vi "Vision.vi"() -> ()   [LabVIEW 2013]
doc: "Use this template to build a standard state machine design pattern. Each state executes code and determines which state to transition to. Contrast this design pattern with the User Interface Event Handler pattern, in which code executes in response to user actions. Contrast this design pattern also with the Queued Message Handler pattern, in which each message handling code can queue zero or more new messages."
uses:
  StateMachineStates 1.ctl
  <vilib>/DAQmx/write.llb/DAQmx Write (Digital Bool 1Line 1Point).vi
  <vilib>/DAQmx/read.llb/DAQmx Read (Digital Bool 1Line 1Point).vi
  <vilib>/DAQmx/read.llb/DAQmx Read (Counter DBL 1Chan 1Samp).vi
  <vilib>/DAQmx/read.llb/DAQmx Read (Counter U32 1Chan 1Samp).vi
  <vilib>/DAQmx/miscellaneous.llb/DAQmx Fill In Error Info.vi
  <vilib>/DAQmx/create/channels.llb/DAQmx Create Channel (CI-Pulse Width).vi
  <vilib>/DAQmx/create/channels.llb/DAQmx Create Channel (CI-Count Edges).vi
panel:
  in  "Dynamic pump power":bool
  out "Set 4":bool[](array[boolean])
  out "Set 3":bool[](array[boolean])
  out "Set 2":bool[](array[boolean])
  out "Set 1":bool[](array[boolean])
  out "Photon time (ms)":dbl format="%.2f"
  in  "Interval (ms)":u32
  out "Repetition":dbl
  in  "Repetitions":dbl=1.0
  out "WP time (ms)":u32
  out "VISA Handle out":refnum<visa-resource-name>="ASRL5::INSTR"
  out "Initializing":bool
  out "Trial mode":T1(ring)
  in  "Frequency of LED trials\nfor Mixed mode":dbl=30.0
  out "Bright trial\nrequested":bool
  out "Observer Ready":bool
  in  "Bright/mixed mode \nLED voltage (V)":dbl=2.6 min=-3.0 max=4.0 format="%.2f"
  in  "Manual voltage (V)":dbl=2.6 format="%.2p"
  in  "GPIB address":string="15"
  in  "Period (ms)":i64=20
  in  "Pulse length (ms)":dbl=50.0
  out "L/R WP":dbl format="%.2f"
  in  "Manually \ninitialize":bool
  in  "COM for WPs":u8=3
  in  "L/R control method":enum16{"Liquid crystal", "Motorized waveplate"}(ring)=enum."Motorized waveplate"
  out "Blocked trial #":i32
  in  "Manual photon #":i32
  out "Photon #":i32
  out "LED Voltage":dbl
  in  "Blocking requirements":cluster{"Value":dbl, " Number":i32}[](array[cluster])
  in  "Manual":bool
  in  "Path":path=path "C:/Users/Lab/Dropbox/Vision software/Data"
  out "Counts 2":u32
  out "Counts 1":u32
  in  "Delay for APDs (ms)":u32=25
  in  "Counter 2":tag="Dev1/ctr1"
  in  "Counter 1":tag="Dev1/ctr0"
  out "Trial #":i32
  in  "Mode":T2(ring)=enum."Mixed"
  in  "Audio":bool=TRUE
  in  "Self-paced":bool
  out "Stimulus":bool
  out "Location Set":bool
  out "Stimulus \nlocation":string
  out "Waiting":bool
  out "Observer Responded":bool
  out "Response \ntime (ms)":dbl
  out "Observer \nchoice":string
  out "Confidence":i32
  in  "stop":bool
  in  "Next Trial":bool
  in  "Create New File":bool
  out "Subject #":string
  # "Settings for Blocking\nand Mixed Mode"
  # "Instructions: Run VI. Enter blocking requirements, then press\nCreate New File. Initialize waveplates if necessary, and set\nhighlighted controls to desired values. Press Next Trial to begin."
  # "Researcher Interface"
  # "Trial Options"
  # "Counter Options\n(same for LED &\ndetector tests)"
  # "Trial Information"
  # "Enter pre-set blocking \nrequirements\nbefore creating a new file."
  # "Troubleshooting"
  # "Photon Options"
  # "LED Options"
  # "Waveplates"
  # "Status"
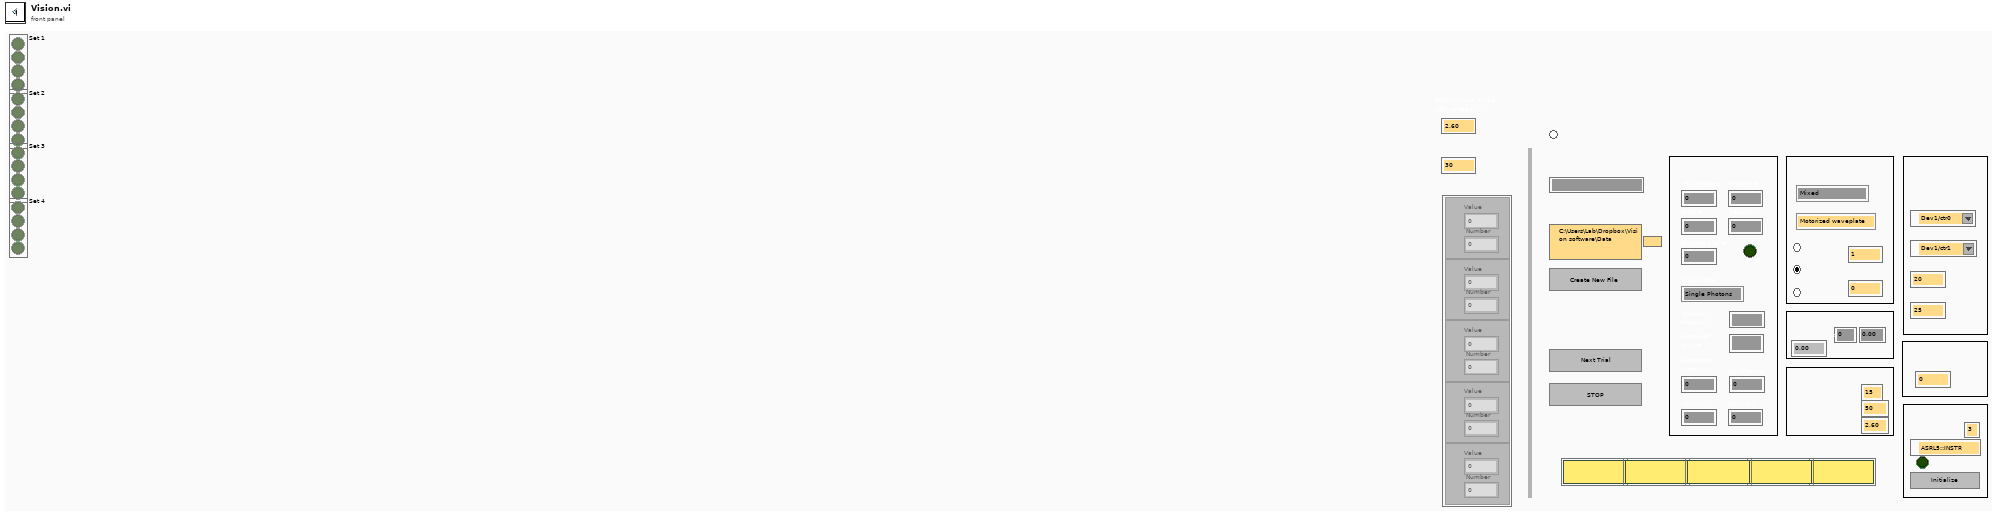
[diagram p1: front panel]
types:
  T1 = enum16{"Single Photons", "Detector Tests", "LED", "Mixed LED"}
  T2 = enum16{"Single Photons", "Detector Tests", "LED", "Mixed"}
  T3 = typedef "StateMachineStates 1.ctl" = enum16{"WaitResearcher", "SetWP", "SetLC", "WaitObserverReady", "Photons", "Detectors", "LED", "WaitObserverResponse", "CleanUp", "Stop"}
  T4 = enum16{"0", "1", "2", "3", "4", "5", "6", "7", "8", "9", "A", "B", "C", "D", "E", "F", "G", "H", "I", "J", "K", "L", "M", "N", "O", "P", "Q", "R", "S", "T", "U", "V", "W", "X", "Y", "Z", "F1", "F2", "F3", "F4", "F5", "F6", "F7", "F8", "F9", "F10", "F11", "F12", "F13", "F14", "F15", "ADD", "BACK", "BACKSLASH", "CAPITAL", "COMMA", "DECIMAL", "DELETE", "DIVIDE", "DOWN", "END", "EQUALS", "ESCAPE", "GRAVE (`)", "HOME", "INSERT", "LBRACKET", "LCONTROL", "LEFT", "L ALT", "LSHIFT", "LWIN", "MINUS", "MULTIPLY", "NEXT", "NUMLOCK", "NUMPAD_0", "NUMPAD_1", "NUMPAD_2", "NUMPAD_3", "NUMPAD_4", "NUMPAD_5", "NUMPAD_6", "NUMPAD_7", "NUMPAD_8", "NUMPAD_9", "PAUSE", "PERIOD", "PRIOR (PG UP)", "RBRACKET", "RCONTROL", "RETURN", "RIGHT", "R ALT", "RSHIFT", "RWIN", "SCROLL", "SEMICOLON", "SLASH", "SPACE", "SUBTRACT", "TAB", "UP", "ENTER (num pad)", "' (quote)"}
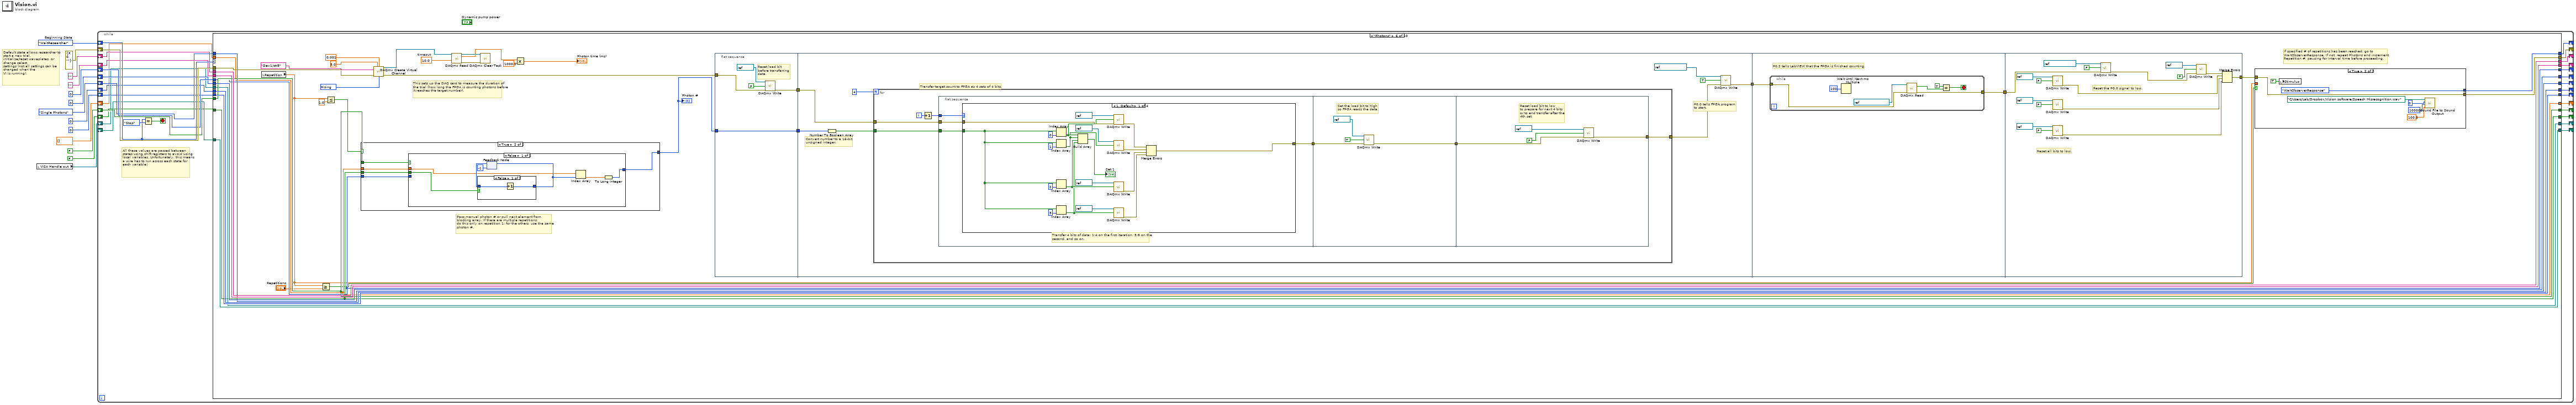
[diagram p0: block diagram]
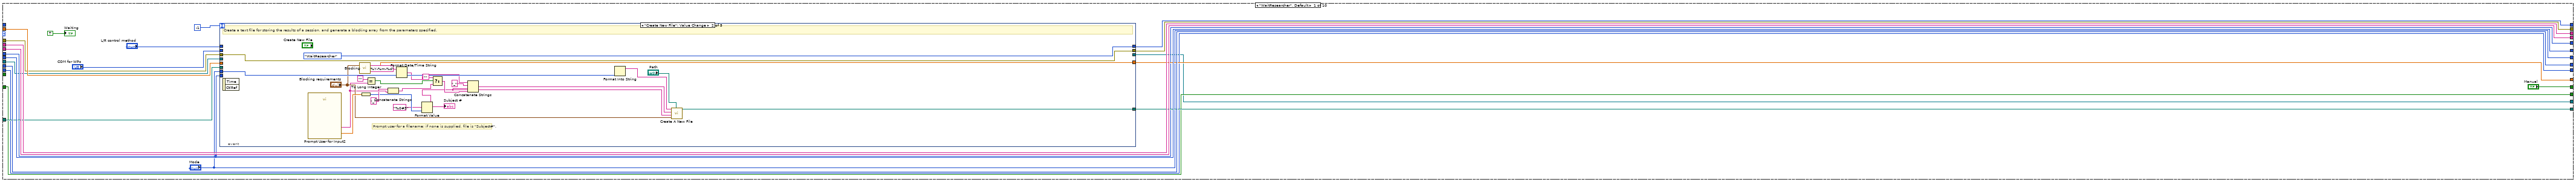
[diagram p2: hidden frame]
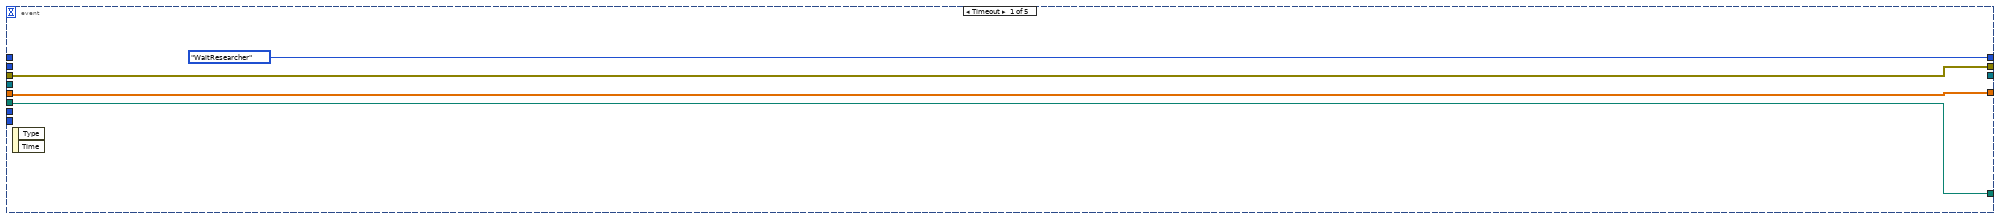
[diagram p3: hidden frame]
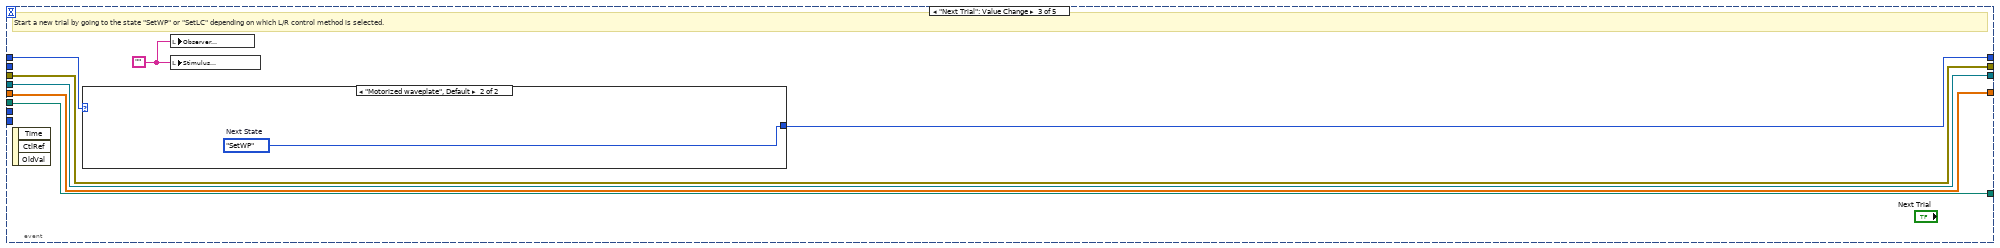
[diagram p4: hidden frame]
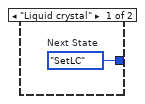
[diagram p5: hidden frame]
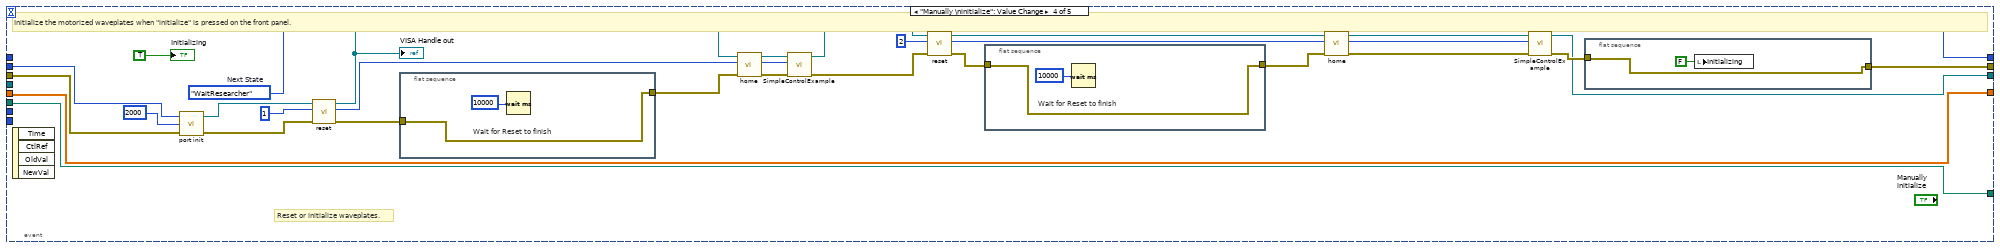
[diagram p6: hidden frame]
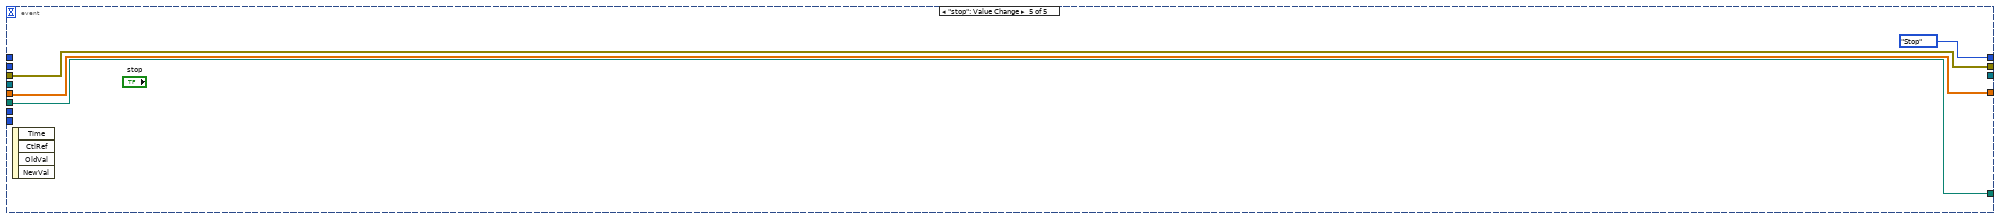
[diagram p7: hidden frame]
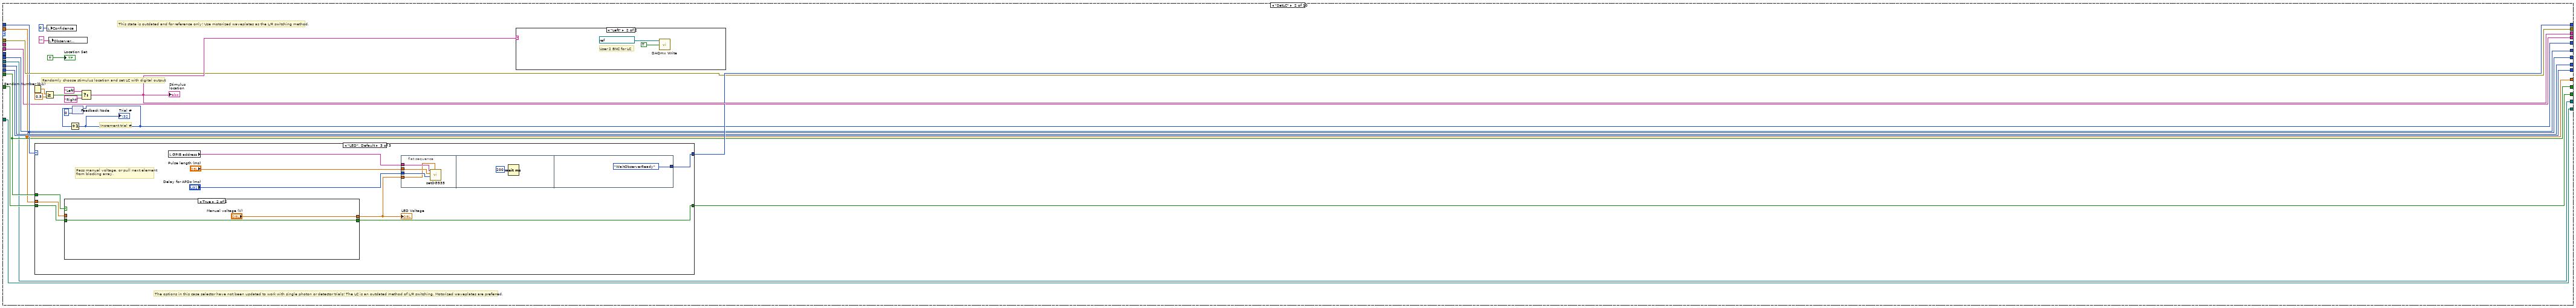
[diagram p8: hidden frame]
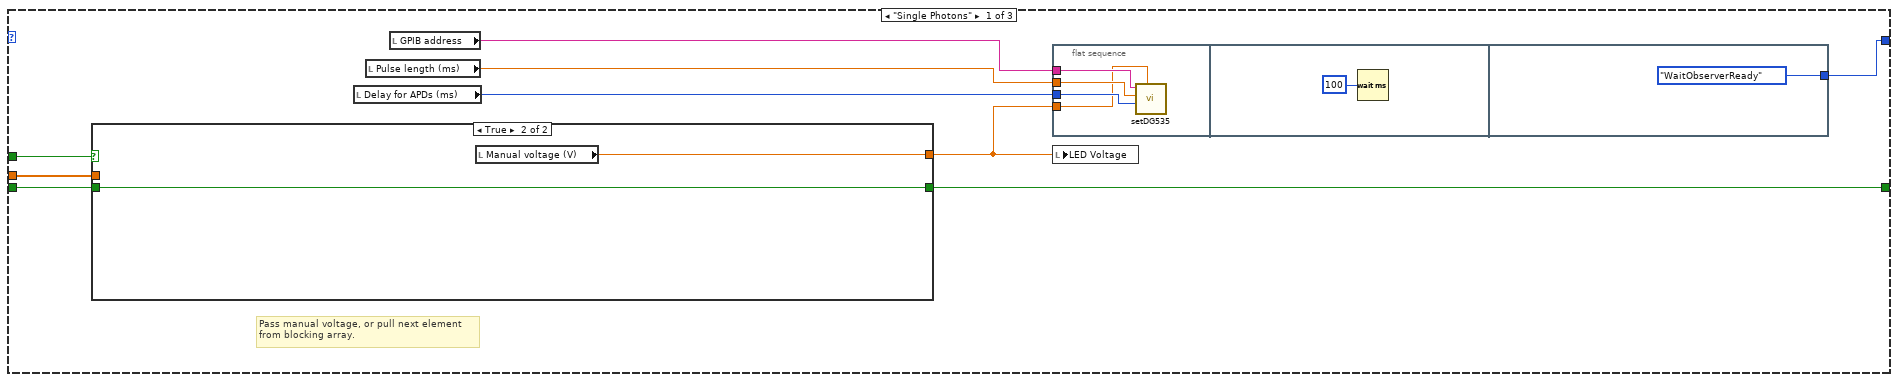
[diagram p9: hidden frame]
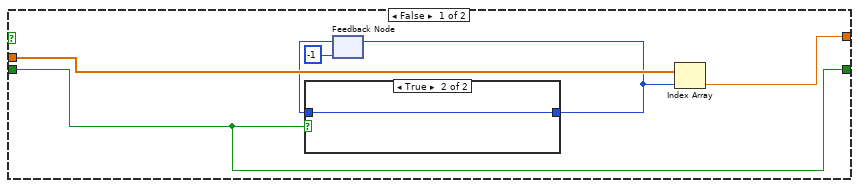
[diagram p10: hidden frame]
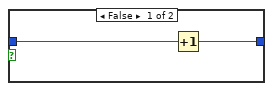
[diagram p11: hidden frame]
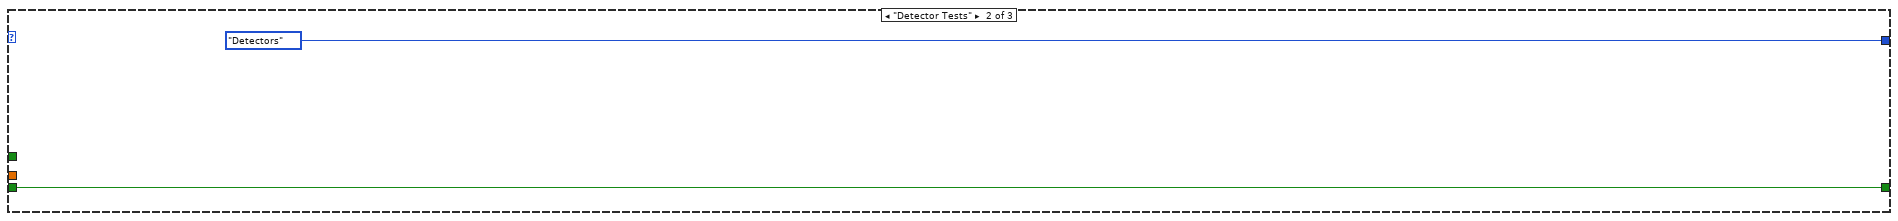
[diagram p12: hidden frame]
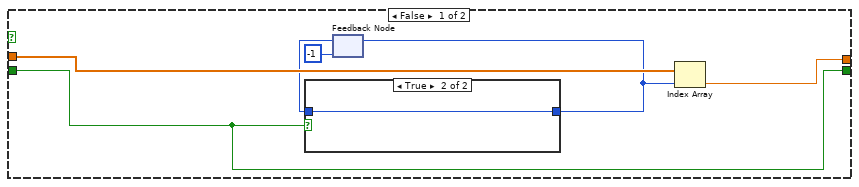
[diagram p13: hidden frame]
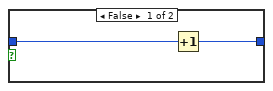
[diagram p14: hidden frame]
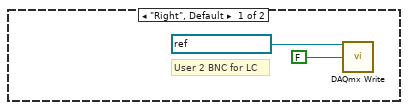
[diagram p15: hidden frame]
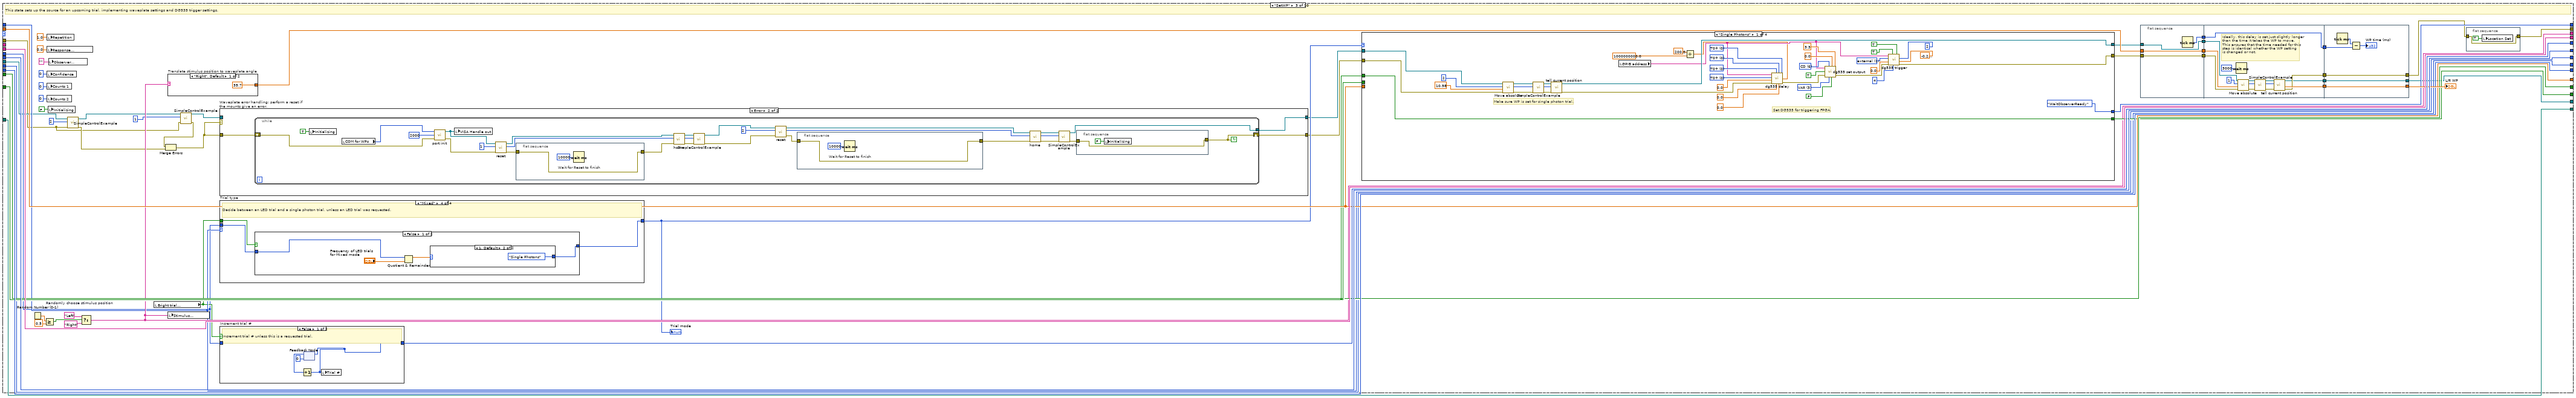
[diagram p16: hidden frame]
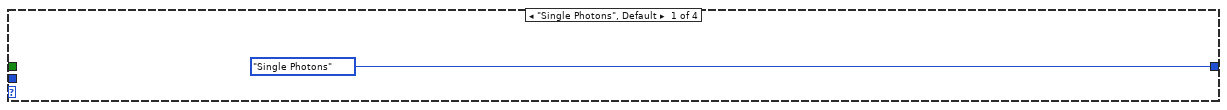
[diagram p19: hidden frame]
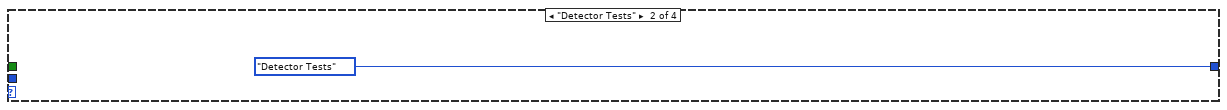
[diagram p20: hidden frame]
diagram:
  w13 = StateMachineStates_1."WaitResearcher"  # Beginning State
  # "Default state allows researcher to start a new trial,\ninitialize/reset waveplates, or change select\nsettings (not all settings can be changed when the\nVI is running)."
  n1 = local read "VISA Handle out"() -> (w1:refnum<visa-resource-name>)
  n2 = while {
    shift-right: [w40] -> _
    shift-left: w13 -> [w41]
    shift-right: [w19] -> _
    shift-left: errorcluster {"status"=FALSE, "code"=0, "source"=""} ("error out") -> [w39]
    shift-right: [w38] -> _
    shift-left: "" -> [w37]
    shift-right: [w36] -> _
    shift-left: "" ("Observer choice") -> [w35]
    shift-right: [w34] -> _
    shift-left: 0 -> [w33]
    shift-right: [w32] -> _
    shift-left: 0 ("Confidence") -> [w31]
    shift-right: [w30] -> _
    shift-left: T2."Single Photons" ("Mode") -> [w29]
    shift-right: [w28] -> _
    shift-left: u32 0 ("Counts 1") -> [w14]
    shift-right: [w27] -> _
    shift-left: u32 0 ("Counts 2") -> [w26]
    shift-right: [w25] -> _
    shift-left: _ -> [w24]
    shift-right: [w23] -> _
    shift-left: dbl[] [] ("Blocking array") -> [w22]
    shift-right: [w21] -> _
    shift-left: FALSE ("Manual") -> [w20]
    shift-right: [w18] -> _
    shift-left: FALSE ("Bright trial\nrequested") -> [w17]
    shift-right: [w16] -> _
    shift-left: w1 -> [w15]
    stop <- w43 stop-if-true
    # "All these values are passed between states using shift registers to avoid using local variables. Unfortunately, this means a wire has to run across each state for each variable!"
    n3 = Equal?(x=w41, y=StateMachineStates_1."Stop" ("States")) -> (x = y?=w43:bool)
    n4 = case shown="\"Photons\"" w41 {
      selector: w41 -> [_ _ _ w527 _ _ _ _ _ _]
      tunnel: [w65 w160 w268 w528 StateMachineStates_1."WaitObserverResponse" ("Next State") w648 w838 w945 w1014 w1092] -> w40
      tunnel: [w50 w157 w267 w516 w607 w638 w824 w949 w997 w1097] -> w19
      tunnel: w39 -> [w51 w157 w226 w517 w593 w625 w840 w949 w991 w1096]
      tunnel: [w64 w161 w261 w531 w608 w651 w846 w951 w1010 w1108] -> w38
      tunnel: w37 -> [w64 _ _ w531 w608 w651 w846 w951 w1010 w1108]
      tunnel: [w63 w145 w278 w530 w611 w650 w819 w946 w1009 w1107] -> w36
      tunnel: w35 -> [w63 w145 w278 w530 w611 w650 _ _ w1009 w1107]
      tunnel: [w53 w151 w276 w529 w598 w641 w841 w950 w1001 w1106] -> w34
      tunnel: w33 -> [w53 _ w242 w529 w598 w641 w841 w950 w1001 w1106]
      tunnel: [w62 w158 w277 w526 w610 w649 w821 w944 w1013 w1105] -> w32
      tunnel: w31 -> [w62 w158 w277 w526 w610 w649 w821 _ w1013 w1105]
      tunnel: ["Mode" w150 w257 w524 w603 w647 w823 w943 w1008 w1104] -> w30
      tunnel: w29 -> [_ w150 w257 w523 w603 w647 w823 w943 w1008 w1104]
      tunnel: [w59 w154 w260 w522 w602 w646 w822 w942 w1006 w1103] -> w28
      tunnel: [w52 w153 w273 w521 w601 w645 w820 w941 w1007 w1102] -> w27
      tunnel: w14 -> [w59 w154 w260 w522 _ w646 _ w942 w1006 w1103]
      tunnel: w26 -> [w52 w153 w273 w521 _ w645 _ w941 w1007 w1102]
      tunnel: [w58 w152 w274 w520 w600 w644 w845 w940 w1005 w1101] -> w25
      tunnel: w24 -> [w57 w152 w274 w520 w600 w644 w845 w940 w1005 w1101]
      tunnel: [w56 w148 w272 w519 w599 w642 w842 w939 w1003 w1100] -> w23
      tunnel: w22 -> [w55 w148 w272 w519 w599 w642 w842 w939 w1003 w1100]
      tunnel: ["Manual" w149 w270 w518 w597 w643 w843 w938 w998 w1099] -> w21
      tunnel: w20 -> [_ w149 w270 w518 w597 w643 w843 w938 w995 w1099]
      tunnel: [w47 w146 w269 w514 w592 w639 w836 w937 w993 w1098] -> w18
      tunnel: w17 -> [w47 w147 w271 w514 w592 w639 w836 w937 _ w1098]
      tunnel: [w46 w142 w254 w513 w591 w640 w835 w936 w992 w1095] -> w16
      tunnel: w15 -> [w44 w142 w235 w513 w591 w640 w835 w936 w992 w1095]
      frame "WaitResearcher", Default {
        n5 = event shown="[1] \"Create New File\": Value Change" {
          selector: _ -> [_ _ _ _ _]
          dyn-events: _ -> [_ _ _ _ _]
          timeout: -1 -> [_ _ _ _ _]
          tunnel: [StateMachineStates_1."WaitResearcher" ("Next State") StateMachineStates_1."WaitResearcher" ("Next State") w96 w131 StateMachineStates_1."Stop" ("Next State")] -> w65
          tunnel: "Mode" -> [_ w88 _ _ _]
          tunnel: [w69 w82 w98 w130 w140] -> w58
          tunnel: w57 -> [w69 _ w98 w130 w140]
          tunnel: [w68 w86 w97 w118 w139] -> w56
          tunnel: w55 -> [w68 _ w97 w118 w139]
          tunnel: w53 -> [_ _ _ _ _]
          tunnel: w51 -> [w67 w81 w94 w119 w138]
          tunnel: [w67 w81 w94 w108 w138] -> w50
          tunnel: "L/R control method" -> [_ _ w95 _ _]
          tunnel: "COM for WPs" -> [_ _ _ w106 _]
          tunnel: [_ _ w93 w104 _] -> w46
          tunnel: w44 -> [_ _ w93 _ _]
          event Timeout {
            n6 = event-data() -> ()  [unwired: 1 in, 2 out]
          }
          event "Create New File": Value Change {
            # "Prompt user for a filename; if none is supplied, file is \"Subject#\"."
            # "Create a text file for storing the results of a session, and generate a blocking array from the parameters specified."
            n7 = event-data() -> ()  [unwired: 1 in, 2 out]
            n8 = call "Prompt User for Input2"() -> ("Subject #"=w91:dbl, "Filename"=w76:string)  [unwired: 16 in, 2 out]
            n9 = call "Blocking.vi"("Blocking requirements"="Blocking requirements") -> ("Blocking array"=w86:dbl[])  [unwired: 2 in]
            n10 = To Long Integer(number=w91) -> (32bit integer=w72:i32)
            n11 = Equal?(x="", y=w76) -> (x = y?=w89:bool)
            n12 = Concatenate Strings("_" ("string"), w76) -> (w79:string)
            n13 = Format Date/Time String(time format string (%c)="%Y-%m-%d") -> (date/time string=w77:string)  [unwired: 2 in]
            n14 = Format Value(format string="%0#3", value (0)=w72) -> (output string=w71:string)  [unwired: 1 in]
            "Subject #" <- w71
            n15 = Select(t="", s=w89, f=w79) -> (s? t:f=w74:string)
            n16 = Concatenate Strings(w77, "_" ("string"), w71, w74) -> (w83:string)
            n17 = Format Into String(w88) -> (resulting string=w87:string)  [unwired: 3 in, 1 out]
            n18 = call "Create A New File.vi"("Path in"="Path", "Blocking requirements"="Blocking requirements", "Subject #"=w71, "Filename"=w83, "Mode"=w87) -> ("Path out"=w82:path)  [unwired: 6 in]
          }
          event "Next Trial": Value Change {
            w99 = ""
            # "Start a new trial by going to the state \"SetWP\" or \"SetLC\" depending on which L/R control method is selected."
            n19 = event-data() -> ()  [unwired: 1 in, 3 out]
            n20 = case shown="\"Motorized waveplate\", Default" w95 {
              tunnel: [w100 w101] -> w96
              frame "Liquid crystal" {
                w100 = StateMachineStates_1."SetLC"  # Next State
              }
              frame "Motorized waveplate", Default {
                w101 = StateMachineStates_1."SetWP"  # Next State
              }
            }
            n21 = local write "Observer \nchoice"(w99) -> ()
            n22 = local write "Stimulus \nlocation"(w99) -> ()
          }
          event "Manually \ninitialize": Value Change {
            w131 = StateMachineStates_1."WaitResearcher"  # Next State
            # "Reset or initialize waveplates."
            # "Initialize the motorized waveplates when \"initialize\" is pressed on the front panel."
            n23 = event-data() -> ()  [unwired: 1 in, 4 out]
            n24 = call "port init.vi"("error in"=w119, "Timeout (ms)"=u32 2000 ("Timeout (300 ms)"), "SerialPort"=w106) -> ("error out"=w126:errorcluster, "Visa Handle"=w125:refnum<visa-resource-name>)  [unwired: 1 in]
            n25 = call "reset.vi"("error in"=w126, "Axis in"=1, "VISA Handle in"=w125) -> ("error out"=w123:errorcluster, "Axis out"=w124:i32, "VISA Handle out"=w102:refnum<visa-resource-name>)  [unwired: 3 in, 1 out]
            "VISA Handle out" <- w102
            n26 = flat-sequence {
              tunnel: [w136] -> w122
              tunnel: w123 -> [w136]
              frame #0 {
                # "Wait for Reset to finish"
                n27 = Wait (ms)(milliseconds to wait=u32 10000) -> ()  [unwired: 1 out]
              }
            }
            n28 = call "home.vi"("error in"=w122, "Axis in"=w124, "VISA Handle in"=w102) -> ("error out"=w128:errorcluster, "Axis out"=w127:i32, "VISA Handle out"=w129:refnum<visa-resource-name>)  [unwired: 3 in, 1 out]
            n29 = call "SimpleControlExample.vi"("error in"=w128, "Axis in"=w127, "VISA Handle in"=w129) -> ("error out"=w107:errorcluster, "VISA Handle out"=w105:refnum<visa-resource-name>)  [unwired: 3 in, 2 out]
            n30 = call "reset.vi"("error in"=w107, "Axis in"=2, "VISA Handle in"=w105) -> ("error out"=w113:errorcluster, "Axis out"=w114:i32, "VISA Handle out"=w110:refnum<visa-resource-name>)  [unwired: 3 in, 1 out]
            n31 = flat-sequence {
              tunnel: [w134] -> w112
              tunnel: w113 -> [w134]
              frame #0 {
                # "Wait for Reset to finish"
                n32 = Wait (ms)(milliseconds to wait=u32 10000) -> ()  [unwired: 1 out]
              }
            }
            n33 = call "home.vi"("error in"=w112, "Axis in"=w114, "VISA Handle in"=w110) -> ("error out"=w116:errorcluster, "Axis out"=w115:i32, "VISA Handle out"=w117:refnum<visa-resource-name>)  [unwired: 3 in, 1 out]
            n34 = call "SimpleControlExample.vi"("error in"=w116, "Axis in"=w115, "VISA Handle in"=w117) -> ("error out"=w109:errorcluster, "VISA Handle out"=w104:refnum<visa-resource-name>)  [unwired: 3 in, 2 out]
            n35 = flat-sequence {
              tunnel: w109 -> [w133]
              tunnel: [w133] -> w108
              frame #0 {
                n36 = local write "Initializing"(FALSE ("Initializing waveplates")) -> ()
              }
            }
            "Initializing" <- TRUE ("Initializing waveplates")
          }
          event "stop": Value Change {
            n37 = event-data() -> ()  [unwired: 1 in, 4 out]
          }
        }
        "Waiting" <- TRUE ("Waiting")
      }
      frame "SetLC" {
        # "This state is outdated and for reference only! Use motorized waveplates as the L/R switching method."
        # "The options in this case selector have not been updated to work with single photon or detector trials! The LC is an outdated method of L/R switching. Motorized waveplates are preferred."
        # "Randomly choose stimulus location and set LC with digital output"
        # "Increment trial #"
        n38 = Random Number (0-1)() -> (number: 0 to 1=w166:dbl)
        n39 = case shown="\"LED\", Default" w150 {
          tunnel: [w172 StateMachineStates_1."Detectors" ("Next State") w197] -> w160
          tunnel: w149 -> [w175 _ w203]
          tunnel: w148 -> [w174 _ w202]
          tunnel: w147 -> [w171 w193 w196]
          tunnel: [w170 w193 w195] -> w146
          frame "Single Photons" {
            # "Pass manual voltage, or pull next element\nfrom blocking array."
            n40 = case shown="True" w175 {
              tunnel: [w186 w191] -> w167
              tunnel: w174 -> [w187 _]
              tunnel: w171 -> [w182 w192]
              tunnel: [w182 w192] -> w170
              frame False {
                n41 = feedback #1(-1 ("x+1")) -> (w185:i32)
                n42 = case shown="True" w182 {
                  tunnel: w185 -> [w189 w190]
                  tunnel: [w188 w190] -> w183
                  frame False {
                    n43 = Increment(x=w189) -> (x+1=w188:i32)
                  }
                  frame True {
                  }
                }
                n44 = feedback-in #1(w183) -> ()
                n45 = Index Array(array=w187, index=w183) -> (element=w186:dbl)
              }
              frame True {
                n46 = local read "Manual voltage (V)"() -> (w191:dbl)
              }
            }
            n47 = local read "Delay for APDs (ms)"() -> (w169:u32)
            n48 = local read "Pulse length (ms)"() -> (w168:dbl)
            n49 = local read "GPIB address"() -> (w173:string)
            n50 = flat-sequence {
              tunnel: w169 -> [w179]
              tunnel: w173 -> [w178]
              tunnel: w168 -> [w177]
              tunnel: w167 -> [w176]
              tunnel: [StateMachineStates_1."WaitObserverReady" ("Next State")] -> w172
              frame #0 {
                n51 = call "setDG535.vi"("amplitude"=w176, "Delay (ms)"=w179, "Pulse length (ms)"=w177, "GPIB address"=w178) -> ()  [unwired: 7 in, 1 out]
              }
              frame #1 {
                n52 = Wait (ms)(milliseconds to wait=u32 100) -> ()  [unwired: 1 out]
              }
              frame #2 {
              }
            }
            n53 = local write "LED Voltage"(w167) -> ()
          }
          frame "Detector Tests" {
          }
          frame "LED", Default {
            # "Pass manual voltage, or pull next element\nfrom blocking array."
            n54 = case shown="True" w203 {
              tunnel: [w214 "Manual voltage (V)"] -> w198
              tunnel: w202 -> [w215 _]
              tunnel: w196 -> [w210 w219]
              tunnel: [w210 w219] -> w195
              frame False {
                n55 = feedback #2(-1 ("x+1")) -> (w213:i32)
                n56 = case shown="True" w210 {
                  tunnel: w213 -> [w217 w218]
                  tunnel: [w216 w218] -> w211
                  frame False {
                    n57 = Increment(x=w217) -> (x+1=w216:i32)
                  }
                  frame True {
                  }
                }
                n58 = feedback-in #2(w211) -> ()
                n59 = Index Array(array=w215, index=w211) -> (element=w214:dbl)
              }
              frame True {
              }
            }
            "LED Voltage" <- w198
            n60 = local read "GPIB address"() -> (w200:string)
            n61 = flat-sequence {
              tunnel: "Delay for APDs (ms)" -> [w207]
              tunnel: w200 -> [w206]
              tunnel: "Pulse length (ms)" -> [w205]
              tunnel: w198 -> [w204]
              tunnel: [StateMachineStates_1."WaitObserverReady" ("Next State")] -> w197
              frame #0 {
                n62 = call "setDG535.vi"("amplitude"=w204, "Delay (ms)"=w207, "Pulse length (ms)"=w205, "GPIB address"=w206) -> ()  [unwired: 7 in, 1 out]
              }
              frame #1 {
                n63 = Wait (ms)(milliseconds to wait=u32 200) -> ()  [unwired: 1 out]
              }
              frame #2 {
              }
            }
          }
        }
        n64 = Greater Or Equal?(x=w166, y=0.5) -> (x >= y?=w164:bool)
        n65 = local write "Confidence"(0 ("Confidence")) -> ()
        n66 = local write "Observer \nchoice"("" ("Observer choice")) -> ()
        n67 = feedback #3(0 ("x+1")) -> (w156:i32)
        n68 = Increment(x=w156) -> (x+1=w151:i32)
        "Trial #" <- w151
        n69 = feedback-in #3(w151) -> ()
        n70 = Select(t="Left", s=w164, f="Right") -> (s? t:f=w161:string)
        "Stimulus \nlocation" <- w161
        n71 = case shown="\"Left\"" w161 {
          frame "Right", Default {
            # "User 2 BNC for LC"
            n72 = call-poly <vilib>:"DAQmx Write.vi"("task/channels in"=refnum<k21> "LC_Controller", "data"=FALSE) -> ()  [unwired: 11 in, 3 out]
          }
          frame "Left" {
            # "User 2 BNC for LC"
            n73 = call-poly <vilib>:"DAQmx Write.vi"("task/channels in"=refnum<k21> "LC_Controller", "data"=TRUE) -> ()  [unwired: 11 in, 3 out]
          }
        }
        "Location Set" <- TRUE ("LC Set")
      }
      frame "SetWP" {
        # "This state sets up the source for an upcoming trial, implementing waveplate settings and DG535 trigger settings."
        n74 = Random Number (0-1)() -> (number: 0 to 1=w262:dbl)
        n75 = Greater Or Equal?(x=w262, y=0.5) -> (x >= y?=w264:bool)
        n76 = local write "Repetition"(1.0 ("Repitition #")) -> ()
        n77 = local write "Response \ntime (ms)"(0.0 ("Response \ntime (ms)")) -> ()
        n78 = local write "Confidence"(0 ("Confidence")) -> ()
        n79 = local write "Counts 1"(u32 0 ("Counts 1")) -> ()
        n80 = local write "Counts 2"(u32 0 ("Counts 2")) -> ()
        n81 = local write "Initializing"(FALSE ("Initializing waveplates")) -> ()
        n82 = local write "Observer \nchoice"("" ("Observer \nchoice")) -> ()
        n83 = call "SimpleControlExample.vi"("error in"=w226, "Axis in"=2, "VISA Handle in"=w235) -> ("error out"=w227:errorcluster, "VISA Handle out"=w233:refnum<visa-resource-name>)  [unwired: 3 in, 2 out]
        n84 = Select "Randomly choose stimulus position"(t="Left", s=w264, f="Right") -> (s? t:f=w261:string)
        n85 = local read "Bright trial\nrequested"() -> (w243:bool)
        n86 = case "Translate stimulus position to waveplate angle" shown="\"Right\", Default" w261 {
          tunnel: [35.7 ("New target position (units)") 80.7 ("New target position (units)")] -> w258
          frame "Right", Default {
          }
          frame "Left" {
          }
        }
        n87 = local write "Stimulus \nlocation"(w261) -> ()
        n88 = call "SimpleControlExample.vi"("error in"=w226, "Axis in"=1, "VISA Handle in"=w233) -> ("error out"=w228:errorcluster, "VISA Handle out"=w231:refnum<visa-resource-name>)  [unwired: 3 in, 2 out]
        n89 = Merge Errors(w228, w227) -> (w225:errorcluster)
        n90 = case "Waveplate error handling: perform a reset if the mounts give an error." shown="Error" w225 {
          tunnel: w225 -> [w280 w283]
          tunnel: [w280 w281] -> w229
          tunnel: [w279 w282] -> w230
          tunnel: w231 -> [w279 _]
          frame No Error {
          }
          frame Error {
            n91 = while {
              tunnel: [w286] -> w282
              shift-right: [w284] -> w281
              shift-left: w283 -> [w289]
              stop <- w284 continue-if-true
              n92 = local write "Initializing"(TRUE ("Initializing waveplates")) -> ()
              n93 = local read "COM for WPs"() -> (w288:u8)
              n94 = call "port init.vi"("error in"=w289, "Timeout (ms)"=u32 2000 ("Timeout (300 ms)"), "SerialPort"=w288) -> ("error out"=w307:errorcluster, "Visa Handle"=w287:refnum<visa-resource-name>)  [unwired: 1 in]
              n95 = local write "VISA Handle out"(w287) -> ()
              n96 = call "reset.vi"("error in"=w307, "Axis in"=1, "VISA Handle in"=w287) -> ("error out"=w305:errorcluster, "Axis out"=w306:i32, "VISA Handle out"=w290:refnum<visa-resource-name>)  [unwired: 3 in, 1 out]
              n97 = flat-sequence {
                tunnel: [w315] -> w304
                tunnel: w305 -> [w315]
                frame #0 {
                  # "Wait for Reset to finish"
                  n98 = Wait (ms)(milliseconds to wait=u32 10000) -> ()  [unwired: 1 out]
                }
              }
              n99 = call "home.vi"("error in"=w304, "Axis in"=w306, "VISA Handle in"=w290) -> ("error out"=w309:errorcluster, "Axis out"=w308:i32, "VISA Handle out"=w310:refnum<visa-resource-name>)  [unwired: 3 in, 1 out]
              n100 = call "SimpleControlExample.vi"("error in"=w309, "Axis in"=w308, "VISA Handle in"=w310) -> ("error out"=w292:errorcluster, "VISA Handle out"=w291:refnum<visa-resource-name>)  [unwired: 3 in, 2 out]
              n101 = call "reset.vi"("error in"=w292, "Axis in"=2, "VISA Handle in"=w291) -> ("error out"=w297:errorcluster, "Axis out"=w298:i32, "VISA Handle out"=w294:refnum<visa-resource-name>)  [unwired: 3 in, 1 out]
              n102 = flat-sequence {
                tunnel: [w313] -> w296
                tunnel: w297 -> [w313]
                frame #0 {
                  # "Wait for Reset to finish"
                  n103 = Wait (ms)(milliseconds to wait=u32 10000) -> ()  [unwired: 1 out]
                }
              }
              n104 = call "home.vi"("error in"=w296, "Axis in"=w298, "VISA Handle in"=w294) -> ("error out"=w300:errorcluster, "Axis out"=w299:i32, "VISA Handle out"=w301:refnum<visa-resource-name>)  [unwired: 3 in, 1 out]
              n105 = call "SimpleControlExample.vi"("error in"=w300, "Axis in"=w299, "VISA Handle in"=w301) -> ("error out"=w293:errorcluster, "VISA Handle out"=w286:refnum<visa-resource-name>)  [unwired: 3 in, 2 out]
              n106 = flat-sequence {
                tunnel: w293 -> [w312]
                tunnel: [w312] -> w284
                frame #0 {
                  n107 = local write "Initializing"(FALSE ("Initializing waveplates")) -> ()
                }
              }
            }
          }
        }
        n108 = case "Trial type" shown="\"Mixed\"" w257 {
          tunnel: [T1."Single Photons" ("Mode") T1."Detector Tests" ("Mode") T1."LED" ("Mode") w325] -> w256
          tunnel: w242 -> [_ _ _ w326]
          tunnel: w243 -> [_ _ _ w324]
          frame "Single Photons", Default {
          }
          frame "Detector Tests" {
          }
          frame "LED" {
          }
          frame "Mixed" {
            # "Decide between an LED trial and a single photon trial, unless an LED trial was requested."
            n109 = case shown="False" w324 {
              tunnel: w326 -> [w330 _]
              tunnel: [w327 T1."Mixed LED" ("Mode")] -> w325
              frame False {
                n110 = Quotient & Remainder(x=w330, y="Frequency of LED trials\nfor Mixed mode") -> (x-y*floor(x/y)=w328:dbl)  [unwired: 1 out]
                n111 = case shown="1, Default" w328 {
                  tunnel: [T1."Mixed LED" ("Mode") T1."Single Photons" ("Mode")] -> w327
                  frame 0 {
                  }
                  frame 1, Default {
                  }
                }
              }
              frame True {
              }
            }
          }
        }
        "Trial mode" <- w256
        n112 = case "Increment trial #" shown="False" w243 {
          tunnel: [w317 w320] -> w276
          tunnel: w242 -> [_ w320]
          frame False {
            # "Increment trial # unless this is a requested trial."
            n113 = feedback #4(0 ("x+1")) -> (w319:i32)
            n114 = Increment(x=w319) -> (x+1=w317:i32)
            n115 = feedback-in #4(w317) -> ()
            n116 = local write "Trial #"(w317) -> ()
          }
          frame True {
          }
        }
        n117 = case shown="\"Single Photons\"" w256 {
          tunnel: [StateMachineStates_1."WaitObserverReady" ("Next State") StateMachineStates_1."Detectors" ("Next State") w462 w502] -> w268
          tunnel: w270 -> [w403 _ w465 _]
          tunnel: w272 -> [_ _ w464 _]
          tunnel: w271 -> [_ w443 w461 w488]
          tunnel: [w403 w443 w460 w488] -> w269
          tunnel: w229 -> [w395 w435 w449 w492]
          tunnel: [w365 w404 w448 w483] -> w252
          tunnel: w230 -> [w364 w433 w446 w490]
          tunnel: [w393 w432 w445 w489] -> w253
          frame "Single Photons" {
            w381 = u32 1 items=["internal", "external", "single shot", "burst", "line"] ("trigger")
            w383 = 3 items=["TTL", "NIM", "ECL", "VAR"] ("mode")
            w385 = u16 6 items=["T0", "A", "B", "AB", "C", "D", "CD"] ("output")
            w388 = u32 0 items=["T0+", "A+", "B+", "C+"] ("D=")
            w389 = u32 0 items=["T0+", "A+", "B+", "D+"] ("C=")
            w390 = u32 0 items=["T0+", "A+", "C+", "D+"] ("B=")
            w391 = u32 0 items=["T0+", "B+", "C+", "D+"] ("A=")
            # "Set DG535 for triggering FPGA."
            # "Make sure WP is set for single photon trial."
            n118 = call "Move absolute.vi"("error in"=w395, "New target position (units)"=10.98, "Axis in"=2, "VISA Handle in"=w364) -> ("error out"=w397:errorcluster, "Axis out"=w398:i32, "VISA Handle out"=w399:refnum<visa-resource-name>)  [unwired: 2 in, 1 out]
            n119 = call "SimpleControlExample.vi"("error in"=w397, "Axis in"=w398, "VISA Handle in"=w399) -> ("error out"=w400:errorcluster, "Axis out"=w401:i32, "VISA Handle out"=w402:refnum<visa-resource-name>)  [unwired: 3 in, 1 out]
            n120 = call "tell current position.vi"("error in"=w400, "Axis in"=w401, "VISA Handle in"=w402) -> ("error out"=w366:errorcluster, "VISA Handle out"=w393:refnum<visa-resource-name>)  [unwired: 2 in, 3 out]
            n121 = local read "GPIB address"() -> (w373:string)
            n122 = Divide(x=200.0 ("D"), y=1000000000.0) -> (x/y=w367:dbl)
            n123 = call "dg535 delay.vi"("C"=0.0, "D"=w367, "D="=w388, "C="=w389, "B"=0.0 ("C"), "error in"=w366, "A"=0.0 ("D"), "B="=w390, "A="=w391, "GPIB address"=w373) -> ("error out"=w387:errorcluster)
            n124 = call "dg535 set output.vi"("GPIB address"=w373, "output"=w385, "set"=TRUE, "error in"=w387, "mode"=w383, "offset"=0.0, "amplitude"=3.3, "load"=FALSE) -> ("error out"=w374:errorcluster)  [unwired: 1 in]
            n125 = call "dg535 trigger.vi"("external trigger level"=sgl -0.2, "burst count"=2, "trigger slope"=TRUE, "burst period"=4, "input impedance"=TRUE, "error in"=w374, "internal/burst trigger rate"=0.0, "trigger"=w381, "GPIB address"=w373) -> ("error out"=w365:errorcluster)
          }
          frame "Detector Tests" {
            w420 = u32 1 items=["internal", "external", "single shot", "burst", "line"] ("trigger")
            w422 = 3 items=["TTL", "NIM", "ECL", "VAR"] ("mode")
            w424 = u16 6 items=["T0", "A", "B", "AB", "C", "D", "CD"] ("output")
            w427 = u32 0 items=["T0+", "A+", "B+", "C+"] ("D=")
            w428 = u32 0 items=["T0+", "A+", "B+", "D+"] ("C=")
            w429 = u32 0 items=["T0+", "A+", "C+", "D+"] ("B=")
            w430 = u32 0 items=["T0+", "B+", "C+", "D+"] ("A=")
            # "Set DG535 for triggering FPGA."
            # "Make sure WP is set for single photon trial."
            n126 = local read "GPIB address"() -> (w412:string)
            n127 = Divide(x=200.0 ("D"), y=1000000000.0) -> (x/y=w406:dbl)
            n128 = call "Move absolute.vi"("error in"=w435, "New target position (units)"=10.98, "Axis in"=2, "VISA Handle in"=w433) -> ("error out"=w437:errorcluster, "Axis out"=w438:i32, "VISA Handle out"=w439:refnum<visa-resource-name>)  [unwired: 2 in, 1 out]
            n129 = call "SimpleControlExample.vi"("error in"=w437, "Axis in"=w438, "VISA Handle in"=w439) -> ("error out"=w440:errorcluster, "Axis out"=w441:i32, "VISA Handle out"=w442:refnum<visa-resource-name>)  [unwired: 3 in, 1 out]
            n130 = call "tell current position.vi"("error in"=w440, "Axis in"=w441, "VISA Handle in"=w442) -> ("error out"=w405:errorcluster, "VISA Handle out"=w432:refnum<visa-resource-name>)  [unwired: 2 in, 3 out]
            n131 = call "dg535 delay.vi"("C"=0.0, "D"=w406, "D="=w427, "C="=w428, "B"=0.0 ("C"), "error in"=w405, "A"=0.0 ("D"), "B="=w429, "A="=w430, "GPIB address"=w412) -> ("error out"=w426:errorcluster)
            n132 = call "dg535 set output.vi"("GPIB address"=w412, "output"=w424, "set"=TRUE, "error in"=w426, "mode"=w422, "offset"=0.0, "amplitude"=3.3, "load"=FALSE) -> ("error out"=w413:errorcluster)  [unwired: 1 in]
            n133 = call "dg535 trigger.vi"("external trigger level"=sgl -0.45, "burst count"=2, "trigger slope"=TRUE, "burst period"=4, "input impedance"=TRUE, "error in"=w413, "internal/burst trigger rate"=0.0, "trigger"=w420, "GPIB address"=w412) -> ("error out"=w404:errorcluster)
          }
          frame "LED", Default {
            # "Make sure WP is set for LED trial."
            # "Set relevent parameters on DG535 for LED flash."
            # "Pass manual voltage, or pull next element\nfrom blocking array."
            n134 = case shown="False" w465 {
              tunnel: [w476 w481] -> w459
              tunnel: w464 -> [w477 _]
              tunnel: w461 -> [w472 w482]
              tunnel: [w472 w482] -> w460
              frame False {
                n135 = feedback #5(-1 ("x+1")) -> (w475:i32)
                n136 = case shown="True" w472 {
                  tunnel: w475 -> [w479 w480]
                  tunnel: [w478 w480] -> w473
                  frame False {
                    n137 = Increment(x=w479) -> (x+1=w478:i32)
                  }
                  frame True {
                  }
                }
                n138 = feedback-in #5(w473) -> ()
                n139 = Index Array(array=w477, index=w473) -> (element=w476:dbl)
              }
              frame True {
                n140 = local read "Manual voltage (V)"() -> (w481:dbl)
              }
            }
            n141 = local read "Delay for APDs (ms)"() -> (w457:u32)
            n142 = local read "Pulse length (ms)"() -> (w458:dbl)
            n143 = local read "GPIB address"() -> (w463:string)
            n144 = call "Move absolute.vi"("error in"=w449, "New target position (units)"=55.98, "Axis in"=2, "VISA Handle in"=w446) -> ("error out"=w451:errorcluster, "Axis out"=w452:i32, "VISA Handle out"=w453:refnum<visa-resource-name>)  [unwired: 2 in, 1 out]
            n145 = local write "LED Voltage"(w459) -> ()
            n146 = flat-sequence {
              tunnel: w457 -> [w469]
              tunnel: w463 -> [w468]
              tunnel: w458 -> [w467]
              tunnel: w459 -> [w466]
              tunnel: [StateMachineStates_1."WaitObserverReady" ("Next State")] -> w462
              frame #0 {
                n147 = call "setDG535.vi"("amplitude"=w466, "Delay (ms)"=w469, "Pulse length (ms)"=w467, "GPIB address"=w468) -> ()  [unwired: 7 in, 1 out]
              }
              frame #1 {
                n148 = Wait (ms)(milliseconds to wait=u32 100) -> ()  [unwired: 1 out]
              }
              frame #2 {
              }
            }
            n149 = call "SimpleControlExample.vi"("error in"=w451, "Axis in"=w452, "VISA Handle in"=w453) -> ("error out"=w454:errorcluster, "Axis out"=w455:i32, "VISA Handle out"=w456:refnum<visa-resource-name>)  [unwired: 3 in, 1 out]
            n150 = call "tell current position.vi"("error in"=w454, "Axis in"=w455, "VISA Handle in"=w456) -> ("error out"=w448:errorcluster, "VISA Handle out"=w445:refnum<visa-resource-name>)  [unwired: 2 in, 3 out]
          }
          frame "Mixed LED" {
            # "Make sure WP is set for LED trial."
            # "Set relevent parameters on DG535 for LED flash."
            n151 = local read "Delay for APDs (ms)"() -> (w500:u32)
            n152 = call "Move absolute.vi"("error in"=w492, "New target position (units)"=55.98, "Axis in"=2, "VISA Handle in"=w490) -> ("error out"=w494:errorcluster, "Axis out"=w495:i32, "VISA Handle out"=w496:refnum<visa-resource-name>)  [unwired: 2 in, 1 out]
            n153 = local read "Pulse length (ms)"() -> (w501:dbl)
            n154 = local read "GPIB address"() -> (w503:string)
            n155 = call "SimpleControlExample.vi"("error in"=w494, "Axis in"=w495, "VISA Handle in"=w496) -> ("error out"=w497:errorcluster, "Axis out"=w498:i32, "VISA Handle out"=w499:refnum<visa-resource-name>)  [unwired: 3 in, 1 out]
            n156 = local read "Bright/mixed mode \nLED voltage (V)"() -> (w487:dbl)
            n157 = call "tell current position.vi"("error in"=w497, "Axis in"=w498, "VISA Handle in"=w499) -> ("error out"=w486:errorcluster, "VISA Handle out"=w489:refnum<visa-resource-name>)  [unwired: 2 in, 3 out]
            n158 = local write "LED Voltage"(w487) -> ()
            n159 = flat-sequence {
              tunnel: w500 -> [w508]
              tunnel: w503 -> [w507]
              tunnel: w501 -> [w506]
              tunnel: w487 -> [w505]
              tunnel: w486 -> [w504]
              tunnel: [w504] -> w484
              tunnel: [w509] -> w485
              tunnel: w484 -> [w509]
              tunnel: [StateMachineStates_1."WaitObserverReady" ("Next State")] -> w502
              tunnel: [w511] -> w483
              tunnel: w485 -> [w511]
              frame #0 {
                n160 = call "setDG535.vi"("amplitude"=w505, "Delay (ms)"=w508, "Pulse length (ms)"=w506, "GPIB address"=w507) -> ()  [unwired: 7 in, 1 out]
              }
              frame #1 {
                n161 = Wait (ms)(milliseconds to wait=u32 100) -> ()  [unwired: 1 out]
              }
              frame #2 {
              }
            }
          }
        }
        n162 = flat-sequence {
          tunnel: w253 -> [w335]
          tunnel: w258 -> [w336]
          tunnel: w252 -> [w337]
          tunnel: [w337] -> w251
          tunnel: [w336] -> w250
          tunnel: [w335] -> w249
          tunnel: [w334] -> w244
          tunnel: w251 -> [w344]
          tunnel: w250 -> [w341]
          tunnel: w249 -> [w340]
          tunnel: [w345] -> w248
          tunnel: [w343] -> w247
          tunnel: [w339] -> w246
          tunnel: [w338] -> w245
          tunnel: w244 -> [w338]
          tunnel: [w356] -> w254
          tunnel: [w357] -> w259
          tunnel: [w358] -> w275
          tunnel: w248 -> [w358]
          tunnel: w247 -> [w357]
          tunnel: w246 -> [w356]
          tunnel: w245 -> [w355]
          frame #0 {
            n163 = Tick Count (ms)() -> (millisecond timer value=w334:u32)
          }
          frame #1 {
            # "Ideally, this delay is set just slightly longer\nthan the time it takes the WP to move.\nThis ensures that the time needed for this\nstep is identical whether the WP setting\nis changed or not."
            n164 = Wait (ms)(milliseconds to wait=u32 3000) -> ()  [unwired: 1 out]
            n165 = call "Move absolute.vi"("error in"=w344, "New target position (units)"=w341, "Axis in"=1, "VISA Handle in"=w340) -> ("error out"=w347:errorcluster, "Axis out"=w348:i32, "VISA Handle out"=w349:refnum<visa-resource-name>)  [unwired: 2 in, 1 out]
            n166 = call "SimpleControlExample.vi"("error in"=w347, "Axis in"=w348, "VISA Handle in"=w349) -> ("error out"=w350:errorcluster, "Axis out"=w351:i32, "VISA Handle out"=w352:refnum<visa-resource-name>)  [unwired: 3 in, 1 out]
            n167 = call "tell current position.vi"("error in"=w350, "Axis in"=w351, "VISA Handle in"=w352) -> ("error out"=w343:errorcluster, "Current position (units)"=w345:dbl, "VISA Handle out"=w339:refnum<visa-resource-name>)  [unwired: 2 in, 2 out]
          }
          frame #2 {
            n168 = Tick Count (ms)() -> (millisecond timer value=w354:u32)
            n169 = Subtract(x=w354, y=w355) -> (x-y=→"WP time (ms)":u32)
          }
        }
        n170 = flat-sequence {
          tunnel: w259 -> [w361]
          tunnel: [w361] -> w267
          frame #0 {
            n171 = local write "Location Set"(TRUE ("Location Set")) -> ()
          }
        }
        "L/R WP" <- w275
      }
      frame "WaitObserverReady" {
        # "Wait for the observer to trigger the beginning of a trial by pressing the spacebar, then go to a stimulus-producing state determined by \"mode\" on the front panel."
        n172 = flat-sequence {
          tunnel: [w532] -> w525
          tunnel: w517 -> [w532]
          tunnel: "Bright/mixed mode \nLED voltage (V)" -> [w535]
          tunnel: w527 -> [w548]
          tunnel: w525 -> [w546]
          tunnel: w523 -> [w541]
          tunnel: "Bright/mixed mode \nLED voltage (V)" -> [w540]
          tunnel: [w542] -> w516
          tunnel: [w549] -> w528
          tunnel: [w545] -> w524
          frame #0 {
            n173 = local read "LED Voltage"() -> (w534:dbl)
            n174 = Greater Or Equal?(x=w534, y=w535) -> (x >= y?=w533:bool)
            n175 = case shown="True" w533 {
              frame False {
                # "If the LED voltage is NOT greater than or equal to the \"bright\" voltage (defined on the front panel), play the normal sound to indicate that the subject may start the trial."
                n176 = call <vilib>:"Beep.vi"() -> ()  [unwired: 12 in]
              }
              frame True {
                # "If the LED voltage is greater than or equal to the \"bright\" voltage (defined on the front panel), play a special sound to alert the subject to a bright trial."
                n177 = call "Sound File to Sound Output.vi"("Volume"=100.0, "Number of Samples/Iteration"=10000, "Device ID"=u32 0, "File Path"=path "C:/Users/Lab/Dropbox/Vision software/Source/notify_short.wav") -> ()
              }
            }
          }
          frame #1 {
            n178 = call "Query Keyboard.vi"("error in (no error)"=w546, "Stop?"=FALSE) -> ("error out"=w543:errorcluster, "element"=w547:T4)  [unwired: 8 in]
            n179 = case shown="\"NUMPAD_0\"" w547 {
              tunnel: [StateMachineStates_1."WaitObserverReady" ("Next State") w557 w564] -> w549
              tunnel: w548 -> [_ _ _]
              tunnel: [w551 w556 w562] -> w545
              tunnel: w541 -> [w551 w556 w562]
              tunnel: w543 -> [w550 w554 w566]
              tunnel: [w550 w554 w565] -> w542
              tunnel: w540 -> [_ _ w563]
              frame "1", Default {
              }
              frame "SPACE" {
                # "If the subject presses SPACE, move to the appropriate stimulus-producing mode (either Photons, Detectors, or LED)."
                n180 = local read "Trial mode"() -> (w553:T1)
                n181 = case shown="\"Single Photons\"" w553 {
                  tunnel: [w558 w559 w560 w561] -> w557
                  frame "Single Photons" {
                    w558 = StateMachineStates_1."Photons"  # Next State
                  }
                  frame "Detector Tests" {
                    w559 = StateMachineStates_1."Detectors"  # Next State
                  }
                  frame "LED", Default {
                    w560 = StateMachineStates_1."LED"  # Next State
                  }
                  frame "Mixed LED" {
                    w561 = StateMachineStates_1."LED"  # Next State
                  }
                }
                "Observer Ready" <- TRUE ("Observer Ready")
              }
              frame "NUMPAD_0" {
                # "If the subject presses 0, request a bright trial and go back to SetWP."
                n182 = case shown="\"Mixed\"" w562 {
                  tunnel: w566 -> [w567 w569 w574 w589]
                  tunnel: [w567 w569 w573 w589] -> w565
                  tunnel: [StateMachineStates_1."WaitObserverReady" ("Next State") StateMachineStates_1."WaitObserverReady" ("Next State") w572 StateMachineStates_1."SetWP" ("Next State")] -> w564
                  tunnel: w563 -> [_ _ w571 _]
                  frame "Single Photons", Default {
                  }
                  frame "Detector Tests" {
                  }
                  frame "LED" {
                    n183 = flat-sequence {
                      tunnel: w574 -> [w579]
                      tunnel: [w578] -> w576
                      tunnel: w571 -> [w577]
                      tunnel: w576 -> [w584]
                      tunnel: [w584] -> w575
                      tunnel: [w587] -> w573
                      tunnel: w575 -> [w587]
                      tunnel: [StateMachineStates_1."WaitObserverReady" ("Next State")] -> w572
                      frame #0 {
                        n184 = local write "LED Voltage"(w577) -> ()
                        n185 = local read "Delay for APDs (ms)"() -> (w581:u32)
                        n186 = local read "Pulse length (ms)"() -> (w580:dbl)
                        n187 = local read "GPIB address"() -> (w582:string)
                        n188 = call "setDG535.vi"("amplitude"=w577, "error in"=w579, "Delay (ms)"=w581, "Pulse length (ms)"=w580, "GPIB address"=w582) -> ("error out"=w578:errorcluster)  [unwired: 6 in]
                      }
                      frame #1 {
                        n189 = Wait (ms)(milliseconds to wait=u32 100) -> ()  [unwired: 1 out]
                      }
                      frame #2 {
                        "Bright trial\nrequested" <- TRUE ("Requested")
                      }
                    }
                  }
                  frame "Mixed" {
                    n190 = local write "Bright trial\nrequested"(TRUE ("Bright trial\nrequested")) -> ()
                  }
                }
              }
            }
          }
        }
      }
      frame "LED" {
        # "Flash LED while reading out counts from two single-photon detectors."
        n191 = local write "Photon #"(0.0 ("Photon #")) -> ()
        n192 = call "flashLED_DG535andcount.vi"("error in"=w593, "GPIB address"="GPIB address", "Period"="Period (ms)", "Counter 2"="Counter 2", "Counter 1"="Counter 1") -> ("Counts 2"=w601:u32, "Counts 1"=w602:u32, "error out"=w606:errorcluster)  [unwired: 4 in]
        "Counts 1" <- w602
        "Counts 2" <- w601
        n193 = flat-sequence {
          tunnel: w606 -> [w612]
          tunnel: [w612] -> w607
          frame #0 {
            "Stimulus" <- TRUE ("Stimulus")
          }
        }
      }
      frame "Photons" {
        w624 = 10.0  # timeout
        w628 = 10280 items=["Rising"=10280, "Falling"=10171] ("Starting Edge")
        # "This sets up the DAQ card to measure the duration of the trial (how long the FPGA is counting photons before it reaches the target number)."
        # "If specified # of repetitions has been reached, go to\nWaitObserverResponse. If not, repeat Photons and increment\nRepetition #, pausing for Interval time before proceeding."
        # "Pass manual photon # or pull next element from\nblocking array. If there are multiple repetitions,\ndo this only on repetition 1; for the others, use the same\nphoton #."
        n194 = local read "Repetition"() -> (w634:dbl)
        n195 = Greater Or Equal?(x=w634, y="Repetitions") -> (x >= y?=w637:bool)
        n196 = Less Or Equal?(x=w634, y=1.0 ("x")) -> (x <= y?=w635:bool)
        n197 = case shown="True" w635 {
          tunnel: w643 -> [_ w795]
          tunnel: w642 -> [_ w794]
          tunnel: w641 -> [_ w793]
          tunnel: [w790 w792] -> w615
          tunnel: w639 -> [_ w791]
          frame False {
            n198 = local read "Photon #"() -> (w790:i32)
          }
          frame True {
            n199 = case shown="False" w795 {
              tunnel: [w802 "Manual photon #"] -> w792
              tunnel: w794 -> [w797 _]
              tunnel: w793 -> [_ _]
              tunnel: w791 -> [w798 _]
              frame False {
                n200 = feedback #6(-1 ("x+1")) -> (w801:i32)
                n201 = case shown="False" w798 {
                  tunnel: w801 -> [w804 w805]
                  tunnel: [w803 w805] -> w799
                  frame False {
                    n202 = Increment(x=w804) -> (x+1=w803:i32)
                  }
                  frame True {
                  }
                }
                n203 = feedback-in #6(w799) -> ()
                n204 = Index Array(array=w797, index=w799) -> (element=w796:dbl)
                n205 = To Long Integer(number=w796) -> (32bit integer=w802:i32)
              }
              frame True {
              }
            }
          }
        }
        "Photon #" <- w615
        n206 = call-poly <vilib>:"DAQmx Create Virtual Channel.vi"("maximum value"=5.0 ("Maximum Value (sec)"), "minimum value"=0.001 ("Minimum Value (sec)"), "counter"=tag "Dev1/ctr3" ("Physical Channel"), "error in"=w625, "starting edge"=w628) -> ("task out"=w629:refnum<k21>, "error out"=w616:errorcluster)  [unwired: 9 in]
        n207 = call-poly <vilib>:"DAQmx Read.vi"("task/channels in"=w629, "timeout"=w624) -> ("task out"=w627:refnum<k21>, "data"=w622:dbl, "error out"=w626:errorcluster)  [unwired: 11 in]
        n208 = call <vilib>:"DAQmx Clear Task.vi"("task in"=w627, "error in"=w626) -> ()  [unwired: 13 in, 1 out]
        n209 = Multiply(x=w622, y=1000.0) -> (x*y=→"Photon time (ms)":dbl)
        n210 = flat-sequence {
          tunnel: w616 -> [w653]
          tunnel: w615 -> [w656]
          tunnel: [w656] -> w620
          tunnel: [w652] -> w619
          tunnel: [w657] -> w618
          tunnel: w620 -> [w664]
          tunnel: w619 -> [w661]
          tunnel: w618 -> [w765]
          tunnel: [w764] -> w617
          tunnel: [w773] -> w614
          tunnel: w617 -> [w779]
          frame #0 {
            # "Reset load bit\nbefore transferring\ndata."
            n211 = call-poly <vilib>:"DAQmx Write.vi"("task/channels in"=refnum<k21> "BIT5", "data"=FALSE, "error in"=w653) -> ("error out"=w652:errorcluster)  [unwired: 10 in, 2 out]
          }
          frame #1 {
            # "P0.0 tells FPGA program \nto start."
            # "Convert number to a 16-bit\nunsigned integer."
            # "Transfer target count to FPGA as 4 sets of 4 bits."
            n212 = Number To Boolean Array(number=w664) -> (Boolean array=w662:bool[])
            n213 = for {
              N: 4 -> [_]
              tunnel: w662 -> [w668]
              tunnel: w661 -> [w670]
              tunnel: [w665] -> w658
              i -> [w671]
              n214 = Increment(x=w671) -> (x+1=w669:i32)
              n215 = flat-sequence {
                tunnel: w670 -> [w675]
                tunnel: w669 -> [w674]
                tunnel: w668 -> [w673]
                tunnel: [w672] -> w667
                tunnel: w667 -> [w757]
                tunnel: [w756] -> w666
                tunnel: w666 -> [w761]
                tunnel: [w760] -> w665
                frame #0 {
                  # "Transfer 4 bits of data: 1:4 on the first iteration, 5:8 on the\nsecond, and so on."
                  n216 = case shown="1, Default" w674 {
                    tunnel: w673 -> [w683 w703 w723 w743]
                    tunnel: w675 -> [w682 w702 w722 w742]
                    tunnel: [w681 w701 w721 w741] -> w672
                    frame 1, Default {
                      n217 = Index Array(array=w683, index=0) -> (element=w680:bool)
                      n218 = Index Array(array=w683, index=1) -> (element=w679:bool)
                      n219 = Index Array(array=w683, index=2) -> (element=w678:bool)
                      n220 = Index Array(array=w683, index=3) -> (element=w677:bool)
                      n221 = Build Array(w680, w679, w678, w677) -> (→"Set 1":bool[])
                      n222 = call-poly <vilib>:"DAQmx Write.vi"("task/channels in"=refnum<k21> "BIT1", "data"=w680, "error in"=w682) -> ("error out"=w691:errorcluster)  [unwired: 10 in, 2 out]
                      n223 = call-poly <vilib>:"DAQmx Write.vi"("task/channels in"=refnum<k21> "BIT2", "data"=w679) -> ("error out"=w690:errorcluster)  [unwired: 11 in, 2 out]
                      n224 = call-poly <vilib>:"DAQmx Write.vi"("task/channels in"=refnum<k21> "BIT3", "data"=w678) -> ("error out"=w689:errorcluster)  [unwired: 11 in, 2 out]
                      n225 = call-poly <vilib>:"DAQmx Write.vi"("task/channels in"=refnum<k21> "BIT4", "data"=w677) -> ("error out"=w688:errorcluster)  [unwired: 11 in, 2 out]
                      n226 = Merge Errors(w691, w690, w689, w688) -> (w681:errorcluster)
                    }
                    frame 2 {
                      n227 = Index Array(array=w703, index=4) -> (element=w700:bool)
                      n228 = Index Array(array=w703, index=5) -> (element=w699:bool)
                      n229 = Index Array(array=w703, index=6) -> (element=w698:bool)
                      n230 = Index Array(array=w703, index=7) -> (element=w697:bool)
                      n231 = Build Array(w700, w699, w698, w697) -> (→"Set 2":bool[])
                      n232 = call-poly <vilib>:"DAQmx Write.vi"("task/channels in"=refnum<k21> "BIT1", "data"=w700, "error in"=w702) -> ("error out"=w711:errorcluster)  [unwired: 10 in, 2 out]
                      n233 = call-poly <vilib>:"DAQmx Write.vi"("task/channels in"=refnum<k21> "BIT2", "data"=w699) -> ("error out"=w710:errorcluster)  [unwired: 11 in, 2 out]
                      n234 = call-poly <vilib>:"DAQmx Write.vi"("task/channels in"=refnum<k21> "BIT3", "data"=w698) -> ("error out"=w709:errorcluster)  [unwired: 11 in, 2 out]
                      n235 = call-poly <vilib>:"DAQmx Write.vi"("task/channels in"=refnum<k21> "BIT4", "data"=w697) -> ("error out"=w708:errorcluster)  [unwired: 11 in, 2 out]
                      n236 = Merge Errors(w711, w710, w709, w708) -> (w701:errorcluster)
                    }
                    frame 3 {
                      n237 = Index Array(array=w723, index=8) -> (element=w720:bool)
                      n238 = Index Array(array=w723, index=9) -> (element=w719:bool)
                      n239 = Index Array(array=w723, index=10) -> (element=w718:bool)
                      n240 = Index Array(array=w723, index=11) -> (element=w717:bool)
                      n241 = Build Array(w720, w719, w718, w717) -> (→"Set 3":bool[])
                      n242 = call-poly <vilib>:"DAQmx Write.vi"("task/channels in"=refnum<k21> "BIT1", "data"=w720, "error in"=w722) -> ("error out"=w731:errorcluster)  [unwired: 10 in, 2 out]
                      n243 = call-poly <vilib>:"DAQmx Write.vi"("task/channels in"=refnum<k21> "BIT2", "data"=w719) -> ("error out"=w730:errorcluster)  [unwired: 11 in, 2 out]
                      n244 = call-poly <vilib>:"DAQmx Write.vi"("task/channels in"=refnum<k21> "BIT3", "data"=w718) -> ("error out"=w729:errorcluster)  [unwired: 11 in, 2 out]
                      n245 = call-poly <vilib>:"DAQmx Write.vi"("task/channels in"=refnum<k21> "BIT4", "data"=w717) -> ("error out"=w728:errorcluster)  [unwired: 11 in, 2 out]
                      n246 = Merge Errors(w731, w730, w729, w728) -> (w721:errorcluster)
                    }
                    frame 4 {
                      n247 = Index Array(array=w743, index=12) -> (element=w740:bool)
                      n248 = Index Array(array=w743, index=13) -> (element=w739:bool)
                      n249 = Index Array(array=w743, index=14) -> (element=w738:bool)
                      n250 = Index Array(array=w743, index=15) -> (element=w737:bool)
                      n251 = Build Array(w740, w739, w738, w737) -> (→"Set 4":bool[])
                      n252 = call-poly <vilib>:"DAQmx Write.vi"("task/channels in"=refnum<k21> "BIT1", "data"=w740, "error in"=w742) -> ("error out"=w751:errorcluster)  [unwired: 10 in, 2 out]
                      n253 = call-poly <vilib>:"DAQmx Write.vi"("task/channels in"=refnum<k21> "BIT2", "data"=w739) -> ("error out"=w750:errorcluster)  [unwired: 11 in, 2 out]
                      n254 = call-poly <vilib>:"DAQmx Write.vi"("task/channels in"=refnum<k21> "BIT3", "data"=w738) -> ("error out"=w749:errorcluster)  [unwired: 11 in, 2 out]
                      n255 = call-poly <vilib>:"DAQmx Write.vi"("task/channels in"=refnum<k21> "BIT4", "data"=w737) -> ("error out"=w748:errorcluster)  [unwired: 11 in, 2 out]
                      n256 = Merge Errors(w751, w750, w749, w748) -> (w741:errorcluster)
                    }
                  }
                }
                frame #1 {
                  # "Set the load bit to high\nso FPGA reads the data."
                  n257 = call-poly <vilib>:"DAQmx Write.vi"("task/channels in"=refnum<k21> "BIT5", "data"=TRUE, "error in"=w757) -> ("error out"=w756:errorcluster)  [unwired: 10 in, 2 out]
                }
                frame #2 {
                  # "Reset load bit to low\nto prepare for next 4 bits\nor to end transfer after the\n4th set."
                  n258 = call-poly <vilib>:"DAQmx Write.vi"("task/channels in"=refnum<k21> "BIT5", "data"=FALSE, "error in"=w761) -> ("error out"=w760:errorcluster)  [unwired: 10 in, 2 out]
                }
              }
            }
            n259 = call-poly <vilib>:"DAQmx Write.vi"("task/channels in"=refnum<k21> "LaserChannel", "data"=TRUE, "error in"=w658) -> ("error out"=w657:errorcluster)  [unwired: 10 in, 2 out]
          }
          frame #2 {
            # "P0.2 tells LabVIEW that the FPGA is finished counting."
            n260 = while {
              tunnel: w765 -> [w771]
              tunnel: [w770] -> w764
              stop <- w767 stop-if-true
              n261 = Wait Until Next ms Multiple(millisecond multiple=u32 100) -> ()  [unwired: 1 out]
              n262 = call-poly <vilib>:"DAQmx Read.vi"("task/channels in"=refnum<k21> "P02countSignal", "error in"=w771) -> ("data"=w768:bool, "error out"=w770:errorcluster)  [unwired: 11 in, 1 out]
              n263 = Equal?(x=TRUE, y=w768) -> (x = y?=w767:bool)
            }
          }
          frame #3 {
            # "Reset all bits to low."
            # "Reset the P0.0 signal to low."
            n264 = call-poly <vilib>:"DAQmx Write.vi"("task/channels in"=refnum<k21> "BIT2", "data"=FALSE) -> ("error out"=w786:errorcluster)  [unwired: 11 in, 2 out]
            n265 = call-poly <vilib>:"DAQmx Write.vi"("task/channels in"=refnum<k21> "BIT3", "data"=FALSE) -> ("error out"=w785:errorcluster)  [unwired: 11 in, 2 out]
            n266 = call-poly <vilib>:"DAQmx Write.vi"("task/channels in"=refnum<k21> "BIT4", "data"=FALSE) -> ("error out"=w784:errorcluster)  [unwired: 11 in, 2 out]
            n267 = call-poly <vilib>:"DAQmx Write.vi"("task/channels in"=refnum<k21> "LaserChannel", "data"=FALSE, "error in"=w779) -> ("error out"=w778:errorcluster)  [unwired: 10 in, 2 out]
            n268 = call-poly <vilib>:"DAQmx Write.vi"("task/channels in"=refnum<k21> "BIT1", "data"=FALSE, "error in"=w778) -> ("error out"=w787:errorcluster)  [unwired: 10 in, 2 out]
            n269 = Merge Errors(w787, w786, w785, w784) -> (w773:errorcluster)
          }
        }
        n270 = case shown="True" w637 {
          tunnel: [StateMachineStates_1."Photons" ("States") StateMachineStates_1."WaitObserverResponse" ("States")] -> w648
          tunnel: w614 -> [w810 w817]
          tunnel: [w810 w817] -> w638
          tunnel: w634 -> [w809 _]
          frame False {
            n271 = Increment(x=w809) -> (x+1=→"Repetition":dbl)
            n272 = Wait (ms)(milliseconds to wait="Interval (ms)") -> ()  [unwired: 1 out]
          }
          frame True {
            n273 = local write "Stimulus"(TRUE ("Counts Taken")) -> ()
            n274 = call "Sound File to Sound Output.vi"("Volume"=100.0, "Number of Samples/Iteration"=10000, "Device ID"=u32 0, "File Path"=path "C:/Users/Lab/Dropbox/Vision software/Speech Misrecognition.wav") -> ()
          }
        }
      }
      frame "Detectors" {
        # "This state is outdated and non-functional! Needs to be updated to work with new FPGA program. 5/29/14"
        n275 = case shown="False" w843 {
          tunnel: [w929 w935] -> w837
          tunnel: w842 -> [w934 _]
          tunnel: w841 -> [w933 _]
          frame False {
            n276 = Subtract(x=w933, y=1) -> (x-y=w931:i32)
            n277 = Index Array(array=w934, index=w931) -> (element=w930:dbl)
            n278 = To Long Integer(number=w930) -> (32bit integer=w929:i32)
          }
          frame True {
            n279 = local read "Manual photon #"() -> (w935:i32)
          }
        }
        n280 = local write "LED Voltage"(0.0 ("LED Voltage")) -> ()
        n281 = flat-sequence {
          tunnel: [w847] -> w839
          tunnel: w840 -> [w848]
          tunnel: w837 -> [w849]
          tunnel: w839 -> [w855]
          tunnel: [w854] -> w834
          tunnel: [w853] -> w833
          tunnel: [w852] -> w832
          tunnel: w834 -> [w871]
          tunnel: [w871] -> w831
          tunnel: [w868] -> w829
          tunnel: w833 -> [w868]
          tunnel: [w867] -> w827
          tunnel: w832 -> [w867]
          tunnel: w831 -> [w873]
          tunnel: [w872] -> w830
          tunnel: w829 -> [w875]
          tunnel: [w875] -> w828
          tunnel: w827 -> [w874]
          tunnel: [w874] -> w826
          tunnel: w830 -> [w902]
          tunnel: [w896] -> w819
          tunnel: [w909] -> w820
          tunnel: [w908] -> w822
          tunnel: w828 -> [w900]
          tunnel: w826 -> [w899]
          tunnel: [w901] -> w825
          tunnel: [w928] -> w838
          tunnel: [w926] -> w824
          tunnel: w825 -> [w926]
          frame #0 {
            n282 = call "NtoFPGA.vi"("error in"=w848, "number"=w849) -> ("error out"=w847:errorcluster)  [unwired: 3 in]
          }
          frame #1 {
            w862 = 10128 items=["Count Up"=10128, "Count Down"=10124, "Externally Controlled"=10326] ("Count Direction")
            w863 = 10280 items=["Rising"=10280, "Falling"=10171] ("Edge")
            w865 = 10128 items=["Count Up"=10128, "Count Down"=10124, "Externally Controlled"=10326] ("Count Direction")
            w866 = 10280 items=["Rising"=10280, "Falling"=10171] ("Edge")
            n283 = local read "Counter 2"() -> (w850:tag)
            n284 = local read "Counter 1"() -> (w851:tag)
            n285 = call-poly <vilib>:"DAQmx Create Virtual Channel.vi"("initial count"=u32 0 ("Initial Count"), "count direction"=w862, "edge"=w863, "counter"=w851, "error in"=w855) -> ("task out"=w860:refnum<k21>, "error out"=w857:errorcluster)  [unwired: 9 in]
            n286 = call-poly <vilib>:"DAQmx Create Virtual Channel.vi"("initial count"=u32 0 ("Initial Count"), "count direction"=w865, "edge"=w866, "counter"=w850, "error in"=w857) -> ("task out"=w859:refnum<k21>, "error out"=w858:errorcluster)  [unwired: 9 in]
            n287 = call <vilib>:"DAQmx Start Task.vi"("task/channels in"=w859, "error in"=w858) -> ("task out"=w852:refnum<k21>, "error out"=w856:errorcluster)  [unwired: 12 in]
            n288 = call <vilib>:"DAQmx Start Task.vi"("task/channels in"=w860, "error in"=w856) -> ("task out"=w853:refnum<k21>, "error out"=w854:errorcluster)  [unwired: 12 in]
          }
          frame #2 {
            # "User 1/P0.0 for Laser"
            n289 = call-poly <vilib>:"DAQmx Write.vi"("task/channels in"=refnum<k21> "LaserChannel", "data"=TRUE) -> ()  [unwired: 11 in, 3 out]
          }
          frame #3 {
            n290 = while {
              tunnel: w873 -> [w881]
              tunnel: [w880] -> w872
              stop <- w877 stop-if-true
              n291 = Wait Until Next ms Multiple(millisecond multiple=u32 100) -> ()  [unwired: 1 out]
              n292 = call-poly <vilib>:"DAQmx Read.vi"("task/channels in"=refnum<k21> "P02countSignal", "error in"=w881) -> ("data"=w878:bool, "error out"=w880:errorcluster)  [unwired: 11 in, 1 out]
              n293 = Equal?(x=TRUE, y=w878) -> (x = y?=w877:bool)
            }
          }
          frame #4 {
            # "Right"
            # "Left"
            n294 = call-poly <vilib>:"DAQmx Read.vi"("task/channels in"=w899, "error in"=w902) -> ("task out"=w904:refnum<k21>, "data"=w888:u32, "error out"=w903:errorcluster)  [unwired: 11 in]
            n295 = To Unsigned Long Integer(number=w888) -> (unsigned 32bit integer=w909:u32)
            n296 = call-poly <vilib>:"DAQmx Read.vi"("task/channels in"=w900, "error in"=w903) -> ("task out"=w905:refnum<k21>, "data"=w894:u32, "error out"=w906:errorcluster)  [unwired: 11 in]
            n297 = Greater Or Equal?(x=w888, y=u32 1) -> (x >= y?=w885:bool)
            n298 = To Unsigned Long Integer(number=w894) -> (unsigned 32bit integer=w908:u32)
            n299 = call <vilib>:"DAQmx Clear Task.vi"("task in"=w905, "error in"=w906) -> ("error out"=w907:errorcluster)  [unwired: 13 in]
            n300 = Greater Or Equal?(x=w894, y=u32 1) -> (x >= y?=w892:bool)
            n301 = Select(t=u32 1 ("y"), s=w885, f=u32 0 ("y")) -> (s? t:f=w884:u32)
            n302 = call <vilib>:"DAQmx Clear Task.vi"("task in"=w904, "error in"=w907) -> ("error out"=w901:errorcluster)  [unwired: 13 in]
            n303 = Number To Decimal String(number=w884) -> (decimal integer string=w898:string)  [unwired: 1 in]
            n304 = Select(t=u32 1 ("y"), s=w892, f=u32 0 ("y")) -> (s? t:f=w889:u32)
            n305 = call-poly <vilib>:"DAQmx Write.vi"("task/channels in"=refnum<k21> "LaserChannel", "data"=FALSE) -> ()  [unwired: 11 in, 3 out]
            n306 = Number To Decimal String(number=w889) -> (decimal integer string=w897:string)  [unwired: 1 in]
            n307 = Concatenate Strings(w897, w898) -> (w895:string)
            n308 = case shown="\"11\"" w895 {
              tunnel: [w912 "Right" w919 "Left"] -> w896
              frame "00", Default {
                n309 = Random Number (0-1)() -> (number: 0 to 1=w913:dbl)
                n310 = Greater Or Equal?(x=w913, y=0.5) -> (x >= y?=w915:bool)
                n311 = Select(t="Left", s=w915, f="Right") -> (s? t:f=w912:string)
              }
              frame "10" {
              }
              frame "11" {
                n312 = Random Number (0-1)() -> (number: 0 to 1=w920:dbl)
                n313 = Greater Or Equal?(x=w920, y=0.5) -> (x >= y?=w922:bool)
                n314 = Select(t="Left", s=w922, f="Right") -> (s? t:f=w919:string)
              }
              frame "01" {
              }
            }
          }
          frame #5 {
            w928 = StateMachineStates_1."CleanUp"  # Next State
            n315 = local write "Stimulus"(TRUE ("Counts Taken")) -> ()
          }
        }
        n316 = local write "Photon #"(w837) -> ()
        n317 = local write "Counts 2"(w820) -> ()
        n318 = local write "Counts 1"(w822) -> ()
        n319 = local write "Observer \nchoice"(w819) -> ()
      }
      frame "WaitObserverResponse" {
        # "Accept user keyboard input and move to CleanUp phase when the spacebar is pressed."
        n320 = flat-sequence {
          tunnel: [w952] -> w948
          tunnel: [w954] -> w947
          tunnel: w948 -> [w954]
          tunnel: [w986] -> w945
          tunnel: [w980] -> w946
          tunnel: [w981] -> w944
          tunnel: w947 -> [w979]
          frame #0 {
            n321 = Get Date/Time In Seconds() -> (seconds since 1Jan1904=w952:timestamp)
            "Confidence" <- 0 ("Confidence")
          }
          frame #1 {
            n322 = while {
              stop <- w958 stop-if-true
              n323 = call "Query Keyboard.vi"("Stop?"=FALSE) -> ("element"=w956:T4)  [unwired: 9 in, 1 out]
              n324 = local read "Confidence"() -> (w961:i32)
              n325 = case shown="\"J\"..\"L\"" w956 {
                tunnel: ["Left" w967 "Right"] -> w957
                frame "D", "F", "S" {
                }
                frame Default {
                  n326 = local read "Observer \nchoice"() -> (w967:string)
                }
                frame "J".."L" {
                }
              }
              "Observer \nchoice" <- w957
              n327 = case shown="\"SPACE\"" w956 {
                tunnel: [FALSE TRUE] -> w960
                frame "0", Default {
                }
                frame "SPACE" {
                }
              }
              n328 = case shown="Default" w956 {
                tunnel: [0 1 2 3 3 2 1] -> w962
                frame Default {
                }
                frame "S" {
                }
                frame "D" {
                }
                frame "F" {
                }
                frame "J" {
                }
                frame "K" {
                }
                frame "L" {
                }
              }
              n329 = Greater Than 0?(x=w961) -> (x > 0?=w959:bool)
              n330 = And(x=w960, y=w959) -> (x .and. y?=w958:bool)
              n331 = Equal To 0?(x=w962) -> (x = 0?=w964:bool)
              n332 = And(x=w964, y=w959) -> (x .and. y?=w963:bool)
              n333 = Select(t=w961, s=w963, f=w962) -> (s? t:f=w965:i32)
              n334 = local write "Confidence"(w965) -> ()
            }
          }
          frame #2 {
            w986 = StateMachineStates_1."CleanUp"  # Next State
            n335 = Get Date/Time In Seconds() -> (seconds since 1Jan1904=w984:timestamp)
            n336 = local read "Confidence"() -> (w981:i32)
            n337 = Subtract(x=w984, y=w979) -> (x-y=w983:dbl)
            n338 = local read "Observer \nchoice"() -> (w980:string)
            n339 = Multiply(x=w983, y=1000.0) -> (x*y=→"Response \ntime (ms)":dbl)
            "Observer Responded" <- TRUE ("Boolean 3")
          }
        }
      }
      frame "CleanUp" {
        n340 = local read "Trial mode"() -> (w989:T1)
        n341 = local read "Subject #"() -> (w1012:string)
        n342 = case shown="True" "Audio" {
          tunnel: w1010 -> [_ w1082]
          tunnel: w1009 -> [_ w1081]
          frame False {
          }
          frame True {
            # "If audio is enabled, play sound for right or wrong answer."
            n343 = Equal?(x=w1082, y=w1081) -> (x = y?=w1083:bool)
            n344 = case shown="True" w1083 {
              frame False {
                n345 = call "Sound File to Sound Output.vi"("Volume"=100.0, "Number of Samples/Iteration"=10000, "Device ID"=u32 0, "File Path"=path "C:/Users/Lab/Dropbox/Vision software/Source/chord_short.wav") -> ()
              }
              frame True {
                n346 = call "Sound File to Sound Output.vi"("Volume"=100.0, "Number of Samples/Iteration"=10000, "Device ID"=u32 0, "File Path"=path "C:/Users/Lab/Dropbox/Vision software/Source/tada_short.wav") -> ()
              }
            }
          }
        }
        n347 = flat-sequence {
          tunnel: w1013 -> [w1037]
          tunnel: w1012 -> [w1034]
          tunnel: w1010 -> [w1030]
          tunnel: w1009 -> [w1029]
          tunnel: w1007 -> [w1028]
          tunnel: w1006 -> [w1026]
          tunnel: w1005 -> [w1024]
          tunnel: w1001 -> [w1019]
          tunnel: w991 -> [w1018]
          tunnel: [w1018] -> w990
          frame #0 {
            # "Write data from trial to file."
            n348 = Equal?(x=w1030, y=w1029) -> (x = y?=w1044:bool)
            n349 = local read "Photon #"() -> (w1021:i32)
            n350 = local read "Photon time (ms)"() -> (w1017:dbl)
            n351 = local read "LED Voltage"() -> (w1022:dbl)
            n352 = local read "Response \ntime (ms)"() -> (w1033:dbl)
            n353 = Select(t=1.0, s=w1044, f=0.0) -> (s? t:f=w1041:dbl)
            n354 = To Long Integer(number=w1033) -> (32bit integer=w1036:i32)
            n355 = To Long Integer(number=w1041) -> (32bit integer=w1040:i32)
            n356 = Number To Engineering String(2:i16 2 ("width (-)"), 4:w1022) -> (0:w1032:string)  [unwired: 2 in]
            n357 = Number To Decimal String(number=w1019) -> (decimal integer string=w1023:string)  [unwired: 1 in]
            n358 = Number To Decimal String(number=w1021) -> (decimal integer string=w1020:string)  [unwired: 1 in]
            n359 = Number To Decimal String(number=w1036) -> (decimal integer string=w1035:string)  [unwired: 1 in]
            n360 = Number To Decimal String(number=w1040) -> (decimal integer string=w1039:string)  [unwired: 1 in]
            n361 = Number To Decimal String(number=w1028) -> (decimal integer string=w1027:string)  [unwired: 1 in]
            n362 = Number To Decimal String(number=w1026) -> (decimal integer string=w1025:string)  [unwired: 1 in]
            n363 = Number To Decimal String(number=w1037) -> (decimal integer string=w1038:string)  [unwired: 1 in]
            n364 = Number To Decimal String(number=w1017, width (-)=i16 5) -> (decimal integer string=w1016:string)
            n365 = Build Array(w1034, w1023, w1030, w1032, w1020, w1029, w1035, w1038, w1039, w1027, w1025, w1016) -> (w1045:string[])
            n366 = call "Write Data.vi"("Trial Results"=w1045, "base path"=w1024) -> ()  [unwired: 10 in]
          }
        }
        n367 = Array Size(array=w1003) -> (size(s)=w1002:i32)
        n368 = Equal?(x=w989, y=T1."Mixed LED") -> (x = y?=w987:bool)
        n369 = flat-sequence {
          tunnel: w990 -> [w1056]
          tunnel: [w1056] -> w996
          tunnel: w995 -> [w1049]
          tunnel: [w1050] -> w994
          tunnel: [w1047] -> w993
          tunnel: w987 -> [w1046]
          tunnel: [w1060] -> w997
          tunnel: w996 -> [w1060]
          frame #0 {
            # "Increment blocked trial # if not in manual mode or\nan LED trial (mixed mode)."
            n370 = feedback #7(0) -> (w1051:i32)
            n371 = local read "Bright trial\nrequested"() -> (w1047:bool)
            n372 = Compound Arithmetic op=OR(w1047, w1049, w1046) -> (w1048:bool)
            n373 = Select(t=0, s=w1048, f=1) -> (s? t:f=w1054:i32)
            n374 = Add(x=w1051, y=w1054) -> (x+y=w1050:i32)
            "Blocked trial #" <- w1050
            n375 = feedback-in #7(w1050) -> ()
          }
          frame #1 {
            w1059 = FALSE ("LC")
            # "Reset indicators"
            n376 = local write "Photon #"(0 ("Photon #")) -> ()
            n377 = local write "Stimulus"(w1059) -> ()
            n378 = local write "Observer Ready"(w1059) -> ()
            n379 = local write "Location Set"(w1059) -> ()
            n380 = local write "Waiting"(w1059) -> ()
            n381 = local write "Bright trial\nrequested"(w1059) -> ()
            n382 = local write "LED Voltage"(0.0 ("LED Voltage")) -> ()
          }
        }
        n383 = Equal?(x=w1002, y=w994) -> (x = y?=w1000:bool)
        n384 = Not(x=w995) -> (.not. x?=w1004:bool)
        n385 = And(x=w1004, y=w1000) -> (x .and. y?=w999:bool)
        n386 = case shown="False" w999 {
          tunnel: [w1063 w1075] -> w1014
          tunnel: w995 -> [w1061 _]
          tunnel: [w1061 w1074] -> w998
          frame False {
            # "Display a message and\nswitch to manual mode\nif end of blocked trials\nis reached."
            n387 = case shown="True" "Self-paced" {
              tunnel: [w1065 w1070] -> w1063
              frame False {
                n388 = call "Display Message to User"() -> ("OK"=w1064:bool)  [unwired: 10 in, 1 out]
                n389 = case shown="True" w1064 {
                  tunnel: [w1066 w1068] -> w1065
                  frame False {
                    w1066 = StateMachineStates_1."CleanUp"  # Next State
                  }
                  frame True {
                    w1068 = StateMachineStates_1."WaitResearcher"  # Next State
                    n390 = local write "Observer Responded"(FALSE ("Observer Responded")) -> ()
                  }
                }
              }
              frame True {
                # "Skip \"WaitingResearcher\" mode if trials are self-paced."
                n391 = local write "Observer Responded"(FALSE ("Observer Responded")) -> ()
                n392 = local read "L/R control method"() -> (w1069:enum16{"Liquid crystal", "Motorized waveplate"})
                n393 = case shown="\"Motorized waveplate\"" w1069 {
                  tunnel: [w1072 w1073] -> w1070
                  frame "Liquid crystal", Default {
                    w1072 = StateMachineStates_1."SetLC"  # Next State
                  }
                  frame "Motorized waveplate" {
                    w1073 = StateMachineStates_1."SetWP"  # Next State
                  }
                }
              }
            }
          }
          frame True {
            w1074 = TRUE ("Manual")
            n394 = local write "Self-paced"(FALSE ("Self-paced")) -> ()
            n395 = local write "Manual"(w1074) -> ()
            n396 = call "Display Message to User2"() -> ("OK"=w1076:bool)  [unwired: 10 in, 1 out]
            n397 = case shown="True" w1076 {
              tunnel: [w1078 w1080] -> w1075
              frame False {
                w1078 = StateMachineStates_1."CleanUp"  # Next State
              }
              frame True {
                w1080 = StateMachineStates_1."WaitResearcher"  # Next State
                n398 = local write "Observer Responded"(FALSE ("Observer Responded")) -> ()
              }
            }
          }
        }
      }
      frame "Stop" {
        n399 = flat-sequence {
          tunnel: w1096 -> [w1110]
          tunnel: w1095 -> [w1109]
          tunnel: [w1111] -> w1094
          tunnel: w1094 -> [w1113]
          tunnel: [w1113] -> w1093
          tunnel: [w1115] -> w1097
          tunnel: w1093 -> [w1115]
          tunnel: [StateMachineStates_1."Stop" ("Next State")] -> w1092
          frame #0 {
            # "Close waveplate session."
            n400 = call "close.vi"("error in"=w1110, "VISA Handle in"=w1109) -> ("error out"=w1111:errorcluster)  [unwired: 3 in]
          }
          frame #1 {
            w1112 = FALSE ("LC")
            # "Reset indicator lights."
            n401 = local write "Observer Ready"(w1112) -> ()
            n402 = local write "Stimulus"(w1112) -> ()
            n403 = local write "Location Set"(w1112) -> ()
            n404 = local write "Observer Responded"(w1112) -> ()
            n405 = local write "Waiting"(w1112) -> ()
          }
          frame #2 {
          }
        }
      }
    }
  }
